vi "02 HEWH 24 Hour Test SM1.vi"(0 "Equipment":T5={"MW100"="MW100", "AG34970"="A-34972A", "WT210"="A-34972A"}, 2 "Semiphore":T6, 11 "Error In":errorcluster) -> (15 "Error Out":errorcluster)   [LabVIEW 2014]
uses:
  Type Definitions/ChannelSettings.ctl
  <vilib>/Utility/file.llb/Write To Spreadsheet File (string).vi
  Type Definitions/PowerElements.ctl
  Type Definitions/TestedFlowratesScenarios.ctl
  Type Definitions/Intellfaucet Mode.ctl
  Type Definitions/ValveBankPositions.ctl
  Type Definitions/HEWH Error Enumeration.ctl
  Support VIs/Global HEWH.vi
  <vilib>/Analysis/NI_AALBase.lvlib
  <vilib>/Analysis/baseanly.llb/Mean (DBL).vi
  Utility/Labview GEA2 Toolkit v2.1/library/GEA2_Toolkit.lvlib
  Type Definitions/EquipReferences.ctl
  Type Definitions/HEWH Tank Indicator.ctl
  <vilib>/Platform/fileVersionInfo.llb/FileVersionInformation.ctl
  Utility/GEA2 Commands/HEWH/Type Definitions/HEWH_Mode.ctl
  Utility/GEA2 Commands/HEWH/Type Definitions/WaterHeater GEA2 Data.ctl
  Utility/LabVIEW GEA2 Toolkit v2.0/type defs/Button Status.ctl
  Utility/GEA2 Commands/HEWH/Type Definitions/Status Query.ctl
  Utility/GEA2 Commands/HEWH/Type Definitions/Service Error Codes.ctl
panel:
  out "DrawCount 2":i32
  out "Dispense Schedule 2":dbl[](array[numeric])=[10.72, 10.72, 10.72, 10.72, 10.72, 10.72] format="%.2f"
  out "Loop":dbl
  out "deleted portion":dbl[](array[numeric])
  in  "Tab Control 3":enum32{"Page 1", "Page 2"}(tab)
  out "Water Heater GEA2 Data":T1 {"CRC" format="%x"; "Length" format="%x"; "Command" format="%x"; "Destination" format="%x"; "Source" format="%x"}
  in  "Tab Control":enum32{"Page 1", "Page 2"}(tab)
  in  "Time Reset":bool
  in  "Time Update":dbl format="%<%H:%M:%S>t"
  out "Tc Tree Check":dbl[](array[numeric]) format="%.4f"
  out "Serial Data In":string
  in  "IP Agilent":string="192.168.25.2"
  in  "IP MW100":string="192.168.25.4"
  out "Label Array":string[](array[string])
  out "Chanel List":string
  out "Computer Name":string
  in  "Stop Logging":bool
  in  "stop":bool
  out "StopSerial":bool
  out "FileVersionInfo Out":T7
  out "GEA2 Write Setpoints":errorcluster
  out "Calibration File Array":dbl[][](array[numeric])
  out "Flow Rate (GPM)":dbl
  out "Degrees F":dbl
  out "Voltage":dbl=240.0
  out "Number of Records":i32
  in  "Stop Test Seqence":bool
  out "Ver.":string
  out "Log Data":string[][](array[string])
  out "DrawCount":i32
  out "POWER":T8
  out "t*=0":dbl format="%<%H:%M:%S>t"
  out "Elapsed.Time (H:M:S)":dbl format="%<%H:%M:%S>t"
  out "STATUS":string
  in  "Help":bool
  out "Tank Display":T9 {"TC6" format="%.2g"; "TIN" format="%.2g"; "TOUT" format="%.2g"; "Mean" format="%.2f"; "Std Dev" format="%.2f"; "TC5" format="%.2g"; "TC4" format="%.2g"; "TC3" format="%.2g"; "TC2" format="%.2g"; "TC1" format="%.2g"}
  out "Current Draw Start Time":dbl format="%.2f"
  out "First Time":bool=TRUE
  out "Current State":string
  out "MW100":refnum<visa-resource-name>
  in  "Tab Control 2":enum32{"TEST STATUS", "DATA VIEW"}(tab)
  in  "Status Tabl":T10(tab)=enum."External Program Controls"
  in  "Read Config File":bool
  in  "RTDin to Downspout Offset":dbl
  in  "Power Off Time":dbl=82800.0 format="%<%H:%M>t"
  in  "End Log Duration":dbl=3600.0 format="%<%H:%M>t"
  in  "Config Filename":string="HEWH First Hour Rating.ini"
  in  "Num of PreDraws(0-3)":i32=1
  out "GEA2 HyperData":bool
  out "Data Array":string[][](array[string])
  in  "Expansion Tank?":bool
  out "Dispense Times":dbl[](array[numeric])=[0.0, 3600.0, 7200.0, 10800.0, 14400.0, 18000.0] format="%<%H:%M>t"
  out "Dispense Schedule":dbl[](array[numeric])=[10.72, 10.72, 10.72, 10.72, 10.72, 10.72] format="%.2f"
  out "Flow Rate Schedule":dbl[](array[numeric])=[3.0, 3.0, 3.0, 3.0, 3.0, 3.0] format="%.2f"
  out "Temperature Schedule":dbl[](array[numeric])=[58.0, 58.0, 58.0, 58.0, 58.0, 58.0] format="%.2f"
  in  "Cold Water Available?":bool=TRUE
  in  "T3":u32=500
  out "Local?":bool
  out "LAN IP Address":string="192.168.25.3"
  out "Init Complete":bool=TRUE
  in  "T1":u32=1000
  in  "T4":u32=30
  in  "T5":u32=50
  in  "Purge Guard Time(s)":dbl=360.0
  out "PowerON":bool=TRUE
  in  "Sample Per.(s)":dbl=5.0
  in  "Power Off Guard Time20s)":u32=20
  in  "Working File Directory":path=path "c:/work"
  in  "Save File Directory":path=path "c:/data"
  out "FileName":path
  out "Use Agilent?":bool
  out "GEA2 Set Mode":T11=enum."HighDemand"
  out "Set PointOut":u8=140
  in  "Calibration File":path=path "C:/work/CalibrationFile.csv"
  out "Calibration File?":bool
  in  "T2":u32=150
  out "Monitoring Temps Chart":T12(graph)
  out "Tcs 1-6":dbl[](array[numeric])
  in  "Purge Right Now":bool
  out "Downspount Flow":dbl(graph)
  out "Downspout Flow":dbl=3.8899999999999997
  out "Downspout Temp":dbl=76.8
  out "Temp Band(+/- F)":dbl=50.0
  out "Flow rate Adj":dbl=85.11482133995038
  out "Downspount Temp":dbl(graph)
  out "TempAdj":dbl
  out "Failed to Start Count":dbl
  in  "RTD Band":dbl=2.0
  in  "Skip Waiting for Cutout":bool
  in  "mean tank upper lim":dbl=140.0
  in  "meant tank lower lim":dbl=130.0
  out "Temp Range Err":bool=TRUE
  out "mean":dbl format="%0.2f"
  in  "Power Off Check Limit":dbl=20.0
  out "M*-1":dbl
  in  "Skip Waiting for Temp 3":bool
  out "Tcs 1-6, Ave. 3":dbl[](array[numeric])
  out "Temps Chart 2":T13(graph)
  in  "Temp Decline Hystersis":dbl=0.2
  out "T_Ave_Max":dbl
  out "T_Ave":dbl
  out "LastDraw":bool=TRUE
  out "T*Max":dbl
  out "Special Last Draw":bool
  out "Discard Last Draw":bool
  out "T*Ave":dbl
  out "T*min":dbl
  out "Volume(Gal.)":dbl
  in  "Flow Adj":dbl=3.0
  in  "Adj Time":dbl=3.0
  in  "K(0.1)":dbl=0.1
  out "TcDown":dbl
  out "Gal Target":dbl
  out "Drawing":bool=TRUE
  out "RTD Out":cluster{dbl, dbl}[](graph)
  out "Flowmeter":cluster{dbl, dbl}[](graph)
  in  "Skip Draw0":bool
  out "TcDown 0":dbl
  out "FlowMeter During Draw0":cluster{dbl, dbl}[](graph)
  out "RTD Out 0":cluster{dbl, dbl}[](graph)
  out "WattHours":dbl
  out "Total Gallons Drawn":dbl
  out "Error History":string[](array[string])
  out "Com History":string[](array[string])
  out "Test Data":dbl[][](array[numeric])
  out "Executaion Sequence":string[](array[string])
  out "Error Datalogging":errorcluster={"status"=TRUE, "code"=-1073807346, "source"="VISA Read in Gather Test Data.vi"}
  out "Gallons Chart":dbl(graph)
  out "Temps":T12(graph) caption="Waveform Chart"
  out "Watt Chart":T14(graph)
  # "24-HOUR RATING TEST"
  # "For Testing Purposes"
  # "Input HEWH Dispense Schedule. Standard Dispense time is 0-5 hours, 10.72 gallons/dispense @ 3 GPM and 58 Deg F."
  # "Wait for Cutout..."
  # "Input relays don't detect that UE or LE are on, and Power reading <\nCompressor LL (0.35 kW currently)"
  # "WAIT FOR TOP HEATER AND COMP OFF."
  # "T*max is max ave temp"
  # "Record output water temp after 15 secs, and at 5 sec intervals thereafter\nMonitor inlet water temp, must be 58 +/- 2 F\nTerminate draw when output temp = T*max -25F, record T*min"
  # "Terminate draw.  Record Tmin*, Tmax*, Tave* and M*"
  # "(For Last Draw, If after 30 sec, T< last tmin, stop and discard measurements, else continue)"
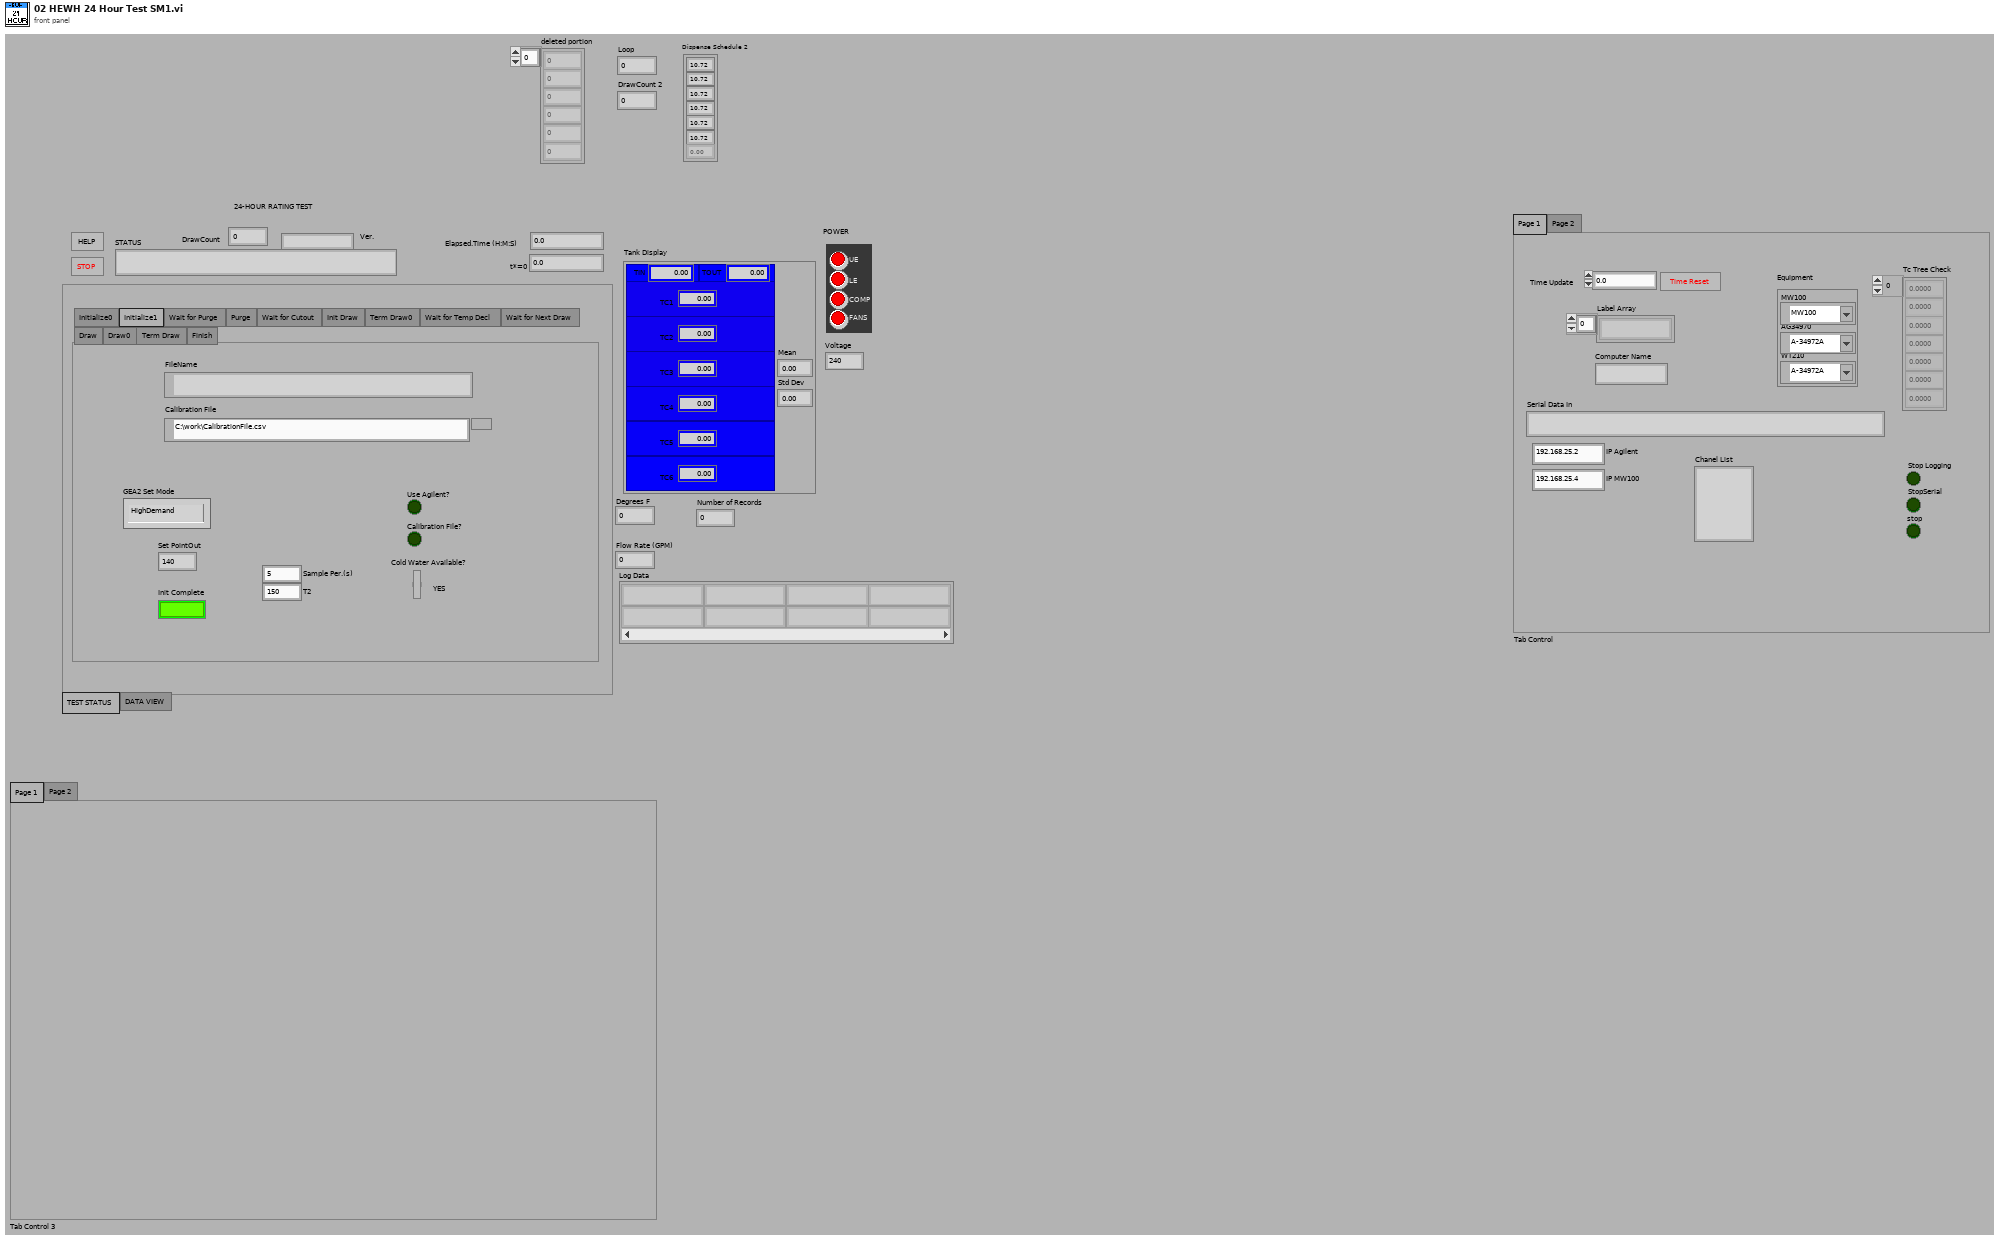
[diagram p1: front panel]
types:
  T1 = typedef "WaterHeater GEA2 Data.ctl" = cluster{"UE - state (1/0 on off)":u8, "LE - state (1/0 on off)":u8, "Comp - state (1/0 on off)":u8, "Fan  - state (1/0 on off)":u8, "Setpoint Deg F":i32, "T2(TankSensor)":dbl, "T3A(EvapIn)":dbl, "T3B(EvapOut)":dbl, "T4(CompressorDischarge)":dbl, "T5(Ambient)":dbl, "Current":dbl, "Voltage (Volts)":u16, "EEV Position (0-480)":u16, "Flow Events (Bit Encoded)":u16, "Heating Control Mode":u16, "Reason for last heating cycle termination":u16, "Reason Data word 1":string, "Reason Data word 2":string, "Reason Data word 3":string, "Reason Data word 4":string, "SW Debug Data":string, "Source":u8, "Destination":u8, "Command":u8, "Length":u8, "CRC":u16, "GEA2 Label Array":string[], " Critical Major SW Version (0-99)":u16, " Critical Minor SW Version (0-99)":u16, "Non Critical Major SW Version (0-99)":u16, "Non Critical Minor SW Version (0-99)":u16, "Software String":string, "GEA2 Data":string[], "Unit System Mode":string, "RQST_CURRENT_PID_SH_TARGET":u16, "RQST_DATA_FROM_DATA_FLASH":string, "RQST_DATA_FROM_Memory":string, "DSM Override Status":string, "IDLB_RESISTANCE":u32, "MODEL NUMBER":string, "MODEL_SELECT_AD_VALUE":u32, "RQST_OVERRIDE_STATUS":string, "PID_PARAMETERS":string[][], "READ_PERSONALITY":u8, "SERIAL_NUMBER":string, "SS_FAULT_COUNTS":string, "STD_ELEC_RANGE":string, "SUPPORTED_MODES":string[][], "T2 Resistance":u32, "T3B Resistance":u32, "T4 Resistance":u32, "T5 Resistance":u32, "Min Set Point (Deg F)":u32, "Max Set Point (Deg F)":u32, "Min Vacation Duration Days":u32, "Max Vacation Duration Days":u32, "Water Capacity (Gallons)":u32, "Button Status":T2, "Status Query":T3, "Service Error Codes":T4, "HEM_KWH_DATA":string[][], "OTHER_FAULT_COUNTS":string[][]}
  T2 = typedef "Button Status.ctl" = cluster{"Switch 1":bool, "Switch 2":bool, "Switch 3":bool, "Switch 4":bool, "Switch 5":bool, "Switch 6":bool, "Switch 7":bool, "Switch 8":bool, "Switch 9":bool, "Switch 10":bool, "Switch 11":bool, "Switch 12":bool, "Switch 13":bool, "Switch 14":bool, "Switch 15":bool, "Switch 16":bool}
  T3 = typedef "Status Query.ctl" = cluster{"Days Remaining (For Std Electric and Vacation)":u8, "Unit Status":string, "Current Tank Temp in Deg F":u8, "Current Setpoint in Deg F":u8, "Filter Status (% used)":u8, "Fallback Status (Fallback heating mode)":string, "Fallback Temp":u8, "\"Set Mode\" Selection":string}
  T4 = typedef "Service Error Codes.ctl" = cluster{"Reserved":bool, "Reserved 1":bool, "Reserved 2":bool, "Reserved 3":bool, "Reserved 4":bool, "Reserved 5":bool, "Reserved 6":bool, "Reserved 7":bool, "DataFlash Fail Status":bool, "Stuck Key Fail Status":bool, "Dry Tank Fail Status":bool, "Miswire Fail Status":bool, "Reserved 8":bool, "Reserved 9":bool, "Reserved 10":bool, "Reserved 11":bool, "UE Fail Status":bool, "LE Fail Status":bool, "Filter Fail Status":bool, "T3A Fail Status":bool, "T3B Fail Status":bool, "T4 Fail Status":bool, "T5 Fail Status":bool, "T2 Fail Status":bool, "SS Cond A Status":bool, "SS Cond B Status":bool, "SS Cond C Status":bool, "SS Cond D Status":bool, "SS Cond E Status":bool, "SS Cond F Status":bool, "SS Fan Status":bool, "CMP Fail Status":bool}
  T5 = typedef "EquipReferences.ctl" = cluster{"MW100":refnum<visa-resource-name>, "AG34970":refnum<visa-resource-name>, "WT210":refnum<visa-resource-name>}
  T6 = typedef "Semaphore RefNum" = refnum<k1>
  T7 = typedef "FileVersionInformation.ctl" = cluster{"FileVersion":string, "ProductName":string, "InternalName":string, "CompanyName":string, "LegalCopyright":string, "FileDescription":string}
  T8 = typedef "PowerElements.ctl" = cluster{"UE":bool, "LE":bool, "COMP":bool, "FANS":bool}
  T9 = typedef "HEWH Tank Indicator.ctl" = cluster{"TC1-D":bool, "TC2-D":bool, "TC3-D":bool, "TC4-D":bool, "TC5-D":bool, "RTD_IN":bool, "RTDOUT":bool, "TC1":dbl, "TC2":dbl, "TC3":dbl, "TC4":dbl, "TC5":dbl, "TIN":dbl, "TOUT":dbl, "Std Dev":dbl, "Mean":dbl, "TC6-D":bool, "TC6":dbl}
  T10 = enum32{"Initialize0", "External Program Controls", "External Program Controls 2", "Program Controls", "Feedback", "Init Draw", "Feedback 2", "Feedback 3", "Feedback 4", "Draw", "Draw0", "Feedback 5", "Feedback 6"}
  T11 = typedef "HEWH_Mode.ctl" = enum16{"Hybrid", "Std Electric", "eHeat", "HighDemand", "Vacation"}
  T12 = cluster{"Tc Tree[0]":dbl, "Tc Tree[1]":dbl, "Tc Tree[2]":dbl, "Tc Tree[3]":dbl, "Tc Tree[4]":dbl, "Tc Tree[5]":dbl}[]
  T13 = cluster{"[0]":dbl, "[1]":dbl, "[2]":dbl, "[3]":dbl, "[4]":dbl, "[5]":dbl, "[6]":dbl}[]
  T14 = cluster{"[0]":dbl, "[1]":dbl, "[2]":dbl, "[3]":dbl, "[4]":dbl, "[5]":dbl}[]
  T15 = typedef "Intellfaucet Mode.ctl" = enum16{"Adjust Temp", "Adjust Flow", "Start Flow", "Stop Flow"}
  T16 = typedef "ValveBankPositions.ctl" = enum16{"Heating", "Purge", "Resting", "Draw"}
  T17 = typedef "TestedFlowratesScenarios.ctl" = enum16{"DRK500,Station1", "DRK375,Lab", "SRK500,Station1,5GPM FR", "DRK375,STATION3,1/2\"HOSE", "DRK500,Station1,downspout", "DRK375,Station3,thruEcocute", "DRK375,Station3,purge", "Build2,2B,Purge", "Global, Purge", "Global, Tank", "DRK250"}
  T18 = typedef "HEWH Error Enumeration.ctl" = enum16{"No Error", "GEA2 Send ACK Mismatch", "GEA2 STX", "GEA2 ETX", "GEA2 CRC Mismatch", "GEA2 ReadACK", "RTD In Range Error", "Fail Mean Tank Temp", "No Flow Config Data Found", "Failed Flow During Purge", "Temp During Purge", "Confirm IF Stop Fail", "Init Draw: TC_1 Out of Range", "Flow = 0 During Draw after 20s"}
  T19 = enum16{"Computation Start", "Computation stop", "Reset Computation", "Clear Computation"}
  T20 = cluster{" Draw Test Condition":enum16{"DRK500,Station1", "DRK375,Lab", "SRK500,Station1,5GPM FR", "DRK500,Station1,downspout"}, "Serial Port Available?":bool, "Cold Water Available?":bool, "TempErLimit":dbl, "Temp Decline Hystersis":dbl, "Target IP Address":string}
  T21 = cluster{"Degree Setting":dbl, "Flow rate setting":dbl, "Tc1 LL":dbl, "Tc1 UL":dbl}
  T22 = cluster{"No Serial  Sample Period(s)":dbl, "T5":u32, "T4":u32, "T1":u32, "T2":u32, "T3":u32}
  T23 = typedef "Cluster Purge Settings.ctl" = cluster{"Temp SettleTimeLimit(S)":dbl, "Steady State Persist Time(mS)":u32, "Purge Min Time":i32, "Flow SettleTimeLimit(S)":dbl, "Flow Adjust Time (3s)":dbl, "Flow Band (+/-GPM)":dbl, "Proportional Control Adjust Rate":dbl}
  T24 = cluster{"PurgreTempLimit":dbl, "Purge Condition TC":enum16{"TC1", "TC2", "TC3", "TC4", "TC5", "TC6"}, "Purgre0TempLim":dbl, "Purge Guard Time(s)":dbl}
  T25 = typedef "GEA2_Toolkit.lvlib/Data In.ctl" = cluster{"Source":u8, "Destination":u8, "Command":u8, "Message":string}
  T26 = typedef "GEA2_Toolkit.lvlib/Data Out.ctl" = cluster{"Source":u8, "Destination":u8, "Command":u8, "Length":u8, "CRC":u16, "Message":string}
  T27 = typedef "Draw Pattern Setup.ctl" = cluster{"Dispense Times":dbl[], "Total Gallons Schedule":dbl[], "Flow Rate Schedule ":dbl[], "Incoming Water Temperature":dbl[], "PreDraw Pattern":dbl[][], "Repeat":bool, "24 Hour PreDraw":T28, "Draw Until?":bool[]}
  T28 = typedef "PreDraw.ctl" = enum16{"Zero Pre-Draws", "One Pre- Draws", "Two Pre-Draws", "Three Pre-Draws", ""}
  T29 = enum16{"Computation Start", "Computation stop", "Reset Computation", "Clear Computation"}[]
  T30 = cluster{"Tc Tree[0]":dbl, "Tc Tree[1]":dbl, "Tc Tree[2]":dbl, "Tc Tree[3]":dbl, "Tc Tree[4]":dbl, "Tc Tree[5]":dbl}
  T31 = cluster{"[0]":dbl, "[1]":dbl, "[2]":dbl, "[3]":dbl, "[4]":dbl, "[5]":dbl, "[6]":dbl}
  T32 = typedef "PowerData.ctl" = cluster{"Voltage (Volts)":dbl, "Current (Amps)":dbl, "Power (Watts)":dbl, "WattHours (Wh)":dbl, "TC Tree (AVG)":dbl, "Flow Rate (GPM)":dbl, "Gallons (Gal)":dbl, "RTD Out (Deg F)":dbl, "TC Down":dbl}
  T33 = typedef "ChannelSettings.ctl" = u32
  T34 = cluster{"[0]":dbl, "[1]":dbl, "[2]":dbl, "[3]":dbl, "[4]":dbl, "[5]":dbl}
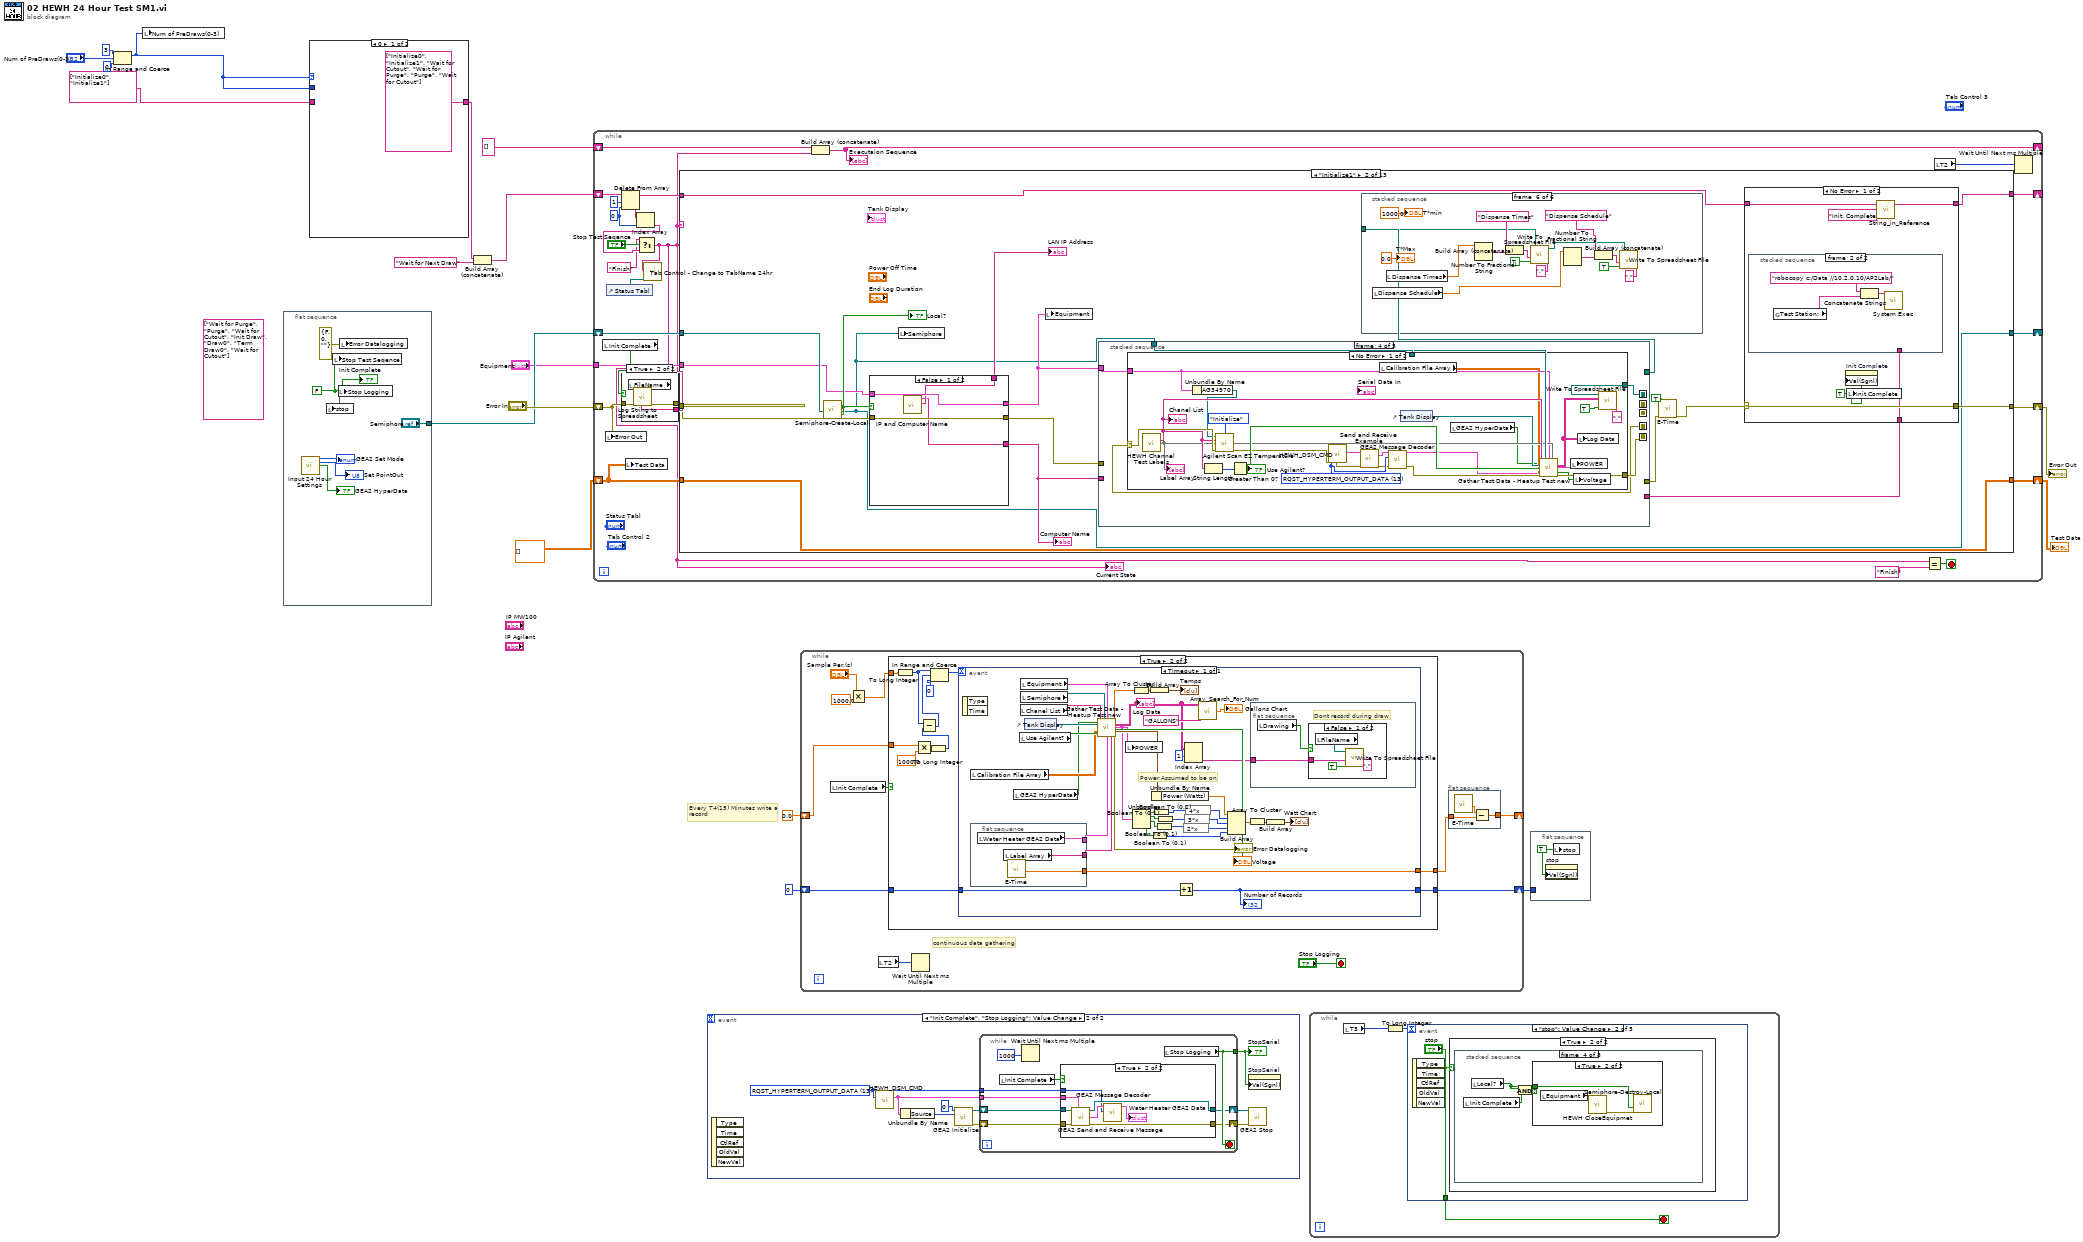
[diagram p0: block diagram]
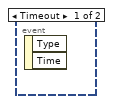
[diagram p2: hidden frame]
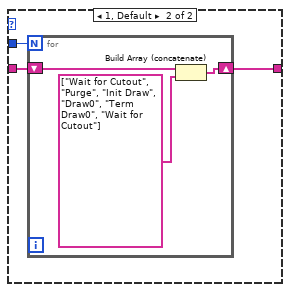
[diagram p4: hidden frame]
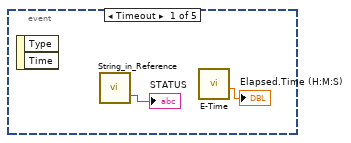
[diagram p5: hidden frame]
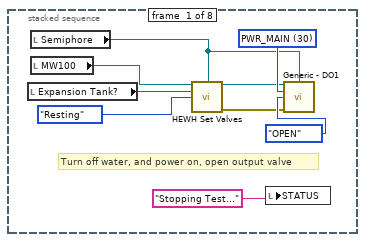
[diagram p7: hidden frame]
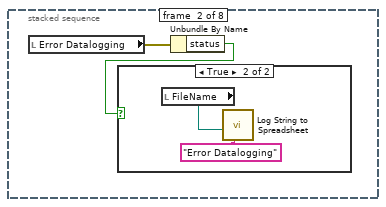
[diagram p8: hidden frame]
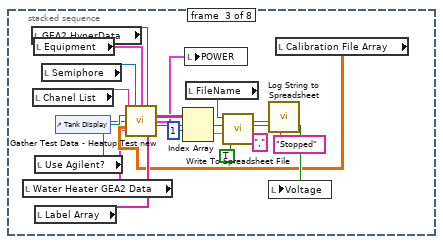
[diagram p10: hidden frame]
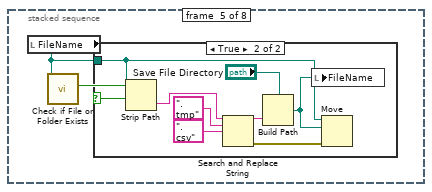
[diagram p12: hidden frame]
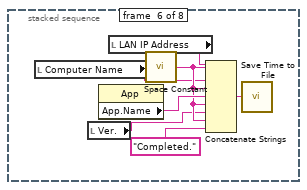
[diagram p14: hidden frame]
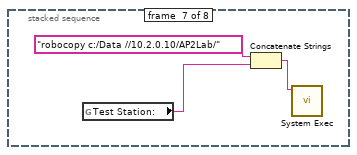
[diagram p15: hidden frame]
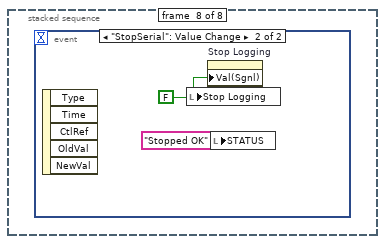
[diagram p16: hidden frame]
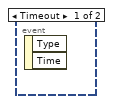
[diagram p17: hidden frame]
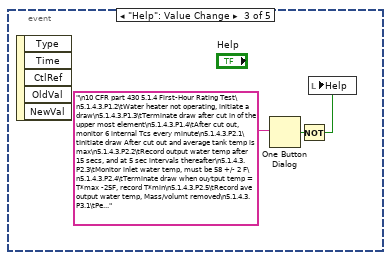
[diagram p18: hidden frame]
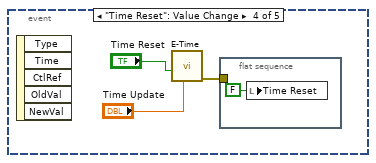
[diagram p19: hidden frame]
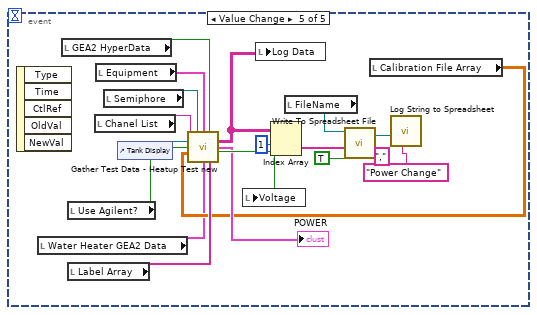
[diagram p20: hidden frame]
diagram:
  (unwired) string[] ["Wait for Purge", "Purge", "Wait for Cutout", "Init Draw", "Draw0", "Term Draw0", "Wait for Cutout"]
  # "Every T4(15) Minutes write a \nrecord"
  n1 = In Range and Coerce(upper limit=3, x="Num of PreDraws(0-3)", lower limit=0) -> (coerced(x)=w4:i32)  [unwired: 1 out]
  n2 = local write "Num of PreDraws(0-3)"(w4) -> ()
  n3 = flat-sequence {
    tunnel: ["Semiphore"] -> w16
    frame #0 {
      w23 = FALSE ("First Time 2")
      n4 = call "Input 24 Hour Settings.vi"() -> ("GEA2 Set Mode Out"=→"GEA2 Set Mode":T11, "Set PointOut"=→"Set PointOut":u8, "GEA2 HyperData Out"=→"GEA2 HyperData":bool)  [unwired: 12 in, 1 out]
      n5 = local write "stop"(w23) -> ()
      n6 = local write "Stop Test Seqence"(w23) -> ()
      n7 = local write "Stop Logging"(w23) -> ()
      n8 = local write "Error Datalogging"(errorcluster {"status"=FALSE, "code"=0, "source"=""} ("errordatalogging")) -> ()
      "Init Complete" <- w23
    }
  }
  n9 = case shown="0" w4 {
    tunnel: [string[] ["Initialize0", "Initialize1", "Wait for Cutout", "Wait for Purge", "Purge", "Wait for Cutout"] w28] -> w10
    tunnel: string[] ["Initialize0", "Initialize1"] -> [_ w27]
    tunnel: w4 -> [_ w26]
    frame 0 {
    }
    frame 1, Default {
      n10 = for {
        N: w26 -> [_]
        shift-right: [w29] -> w28
        shift-left: w27 -> [w31]
        n11 = Build Array (concatenate)(w31, string[] ["Wait for Cutout", "Purge", "Init Draw", "Draw0", "Term Draw0", "Wait for Cutout"]) -> (w29:string[])
      }
    }
  }
  n12 = Build Array (concatenate)(w10, "Wait for Next Draw") -> (w5:string[])
  n13 = while {
    shift-right: [w53] -> _
    shift-left: w5 -> [w56]
    shift-right: [w51] -> w17
    shift-left: "Error In" -> [w39]
    tunnel: "Equipment" -> [w47]
    shift-right: [w46] -> w14
    shift-left: dbl[][] [] -> [w45]
    shift-right: [w44] -> _
    shift-left: w16 -> [w48]
    shift-right: [w40] -> _
    shift-left: string[] [] -> [w41]
    stop <- w50 stop-if-true
    w43 = 0 ("index")
    n14 = local read "Init Complete"() -> (w37:bool)
    n15 = local write "Error Out"(w39) -> ()
    n16 = control-ref of="Status Tabl"() -> (w36:refnum<vi>)
    n17 = Delete From Array(array=w56, length=1, index=w43) -> (deleted portion=w54:string[], array with subset deleted=w52:string[])
    n18 = local write "Test Data"(w45) -> ()
    n19 = Index Array(array=w54, index=w43) -> (element=w34:string)
    n20 = Select(t="Finish" ("y"), s="Stop Test Seqence", f=w34) -> (s? t:f=w33:string)
    "Current State" <- w33
    n21 = case shown="True" w37 {
      tunnel: w39 -> [w57 w60]
      tunnel: [w57 w59] -> w38
      tunnel: w33 -> [_ w58]
      frame False {
      }
      frame True {
        n22 = local read "FileName"() -> (w61:path)
        n23 = call "Log String to Spreadsheet.vi"("String"=w58, "error in (no error)"=w60, "FileName"=w61) -> ("error out"=w59:errorcluster)  [unwired: 8 in]
      }
    }
    n24 = call "Tab Control - Change to TabName 24hr.vi"("Label.Text"=w33, "Status Tabl 3"=w36) -> ()  [unwired: 9 in]
    n25 = case shown="\"Initialize1\"" w33 {
      selector: w33 -> [_ _ _ _ _ _ _ _ _ _ _ _ w1179]
      tunnel: [w70 w113 w297 w375 w432 w553 w625 w691 w705 w886 w1028 w1145 w1194] -> w53
      tunnel: w52 -> [w70 w114 w298 w373 w430 w551 w626 w692 _ w887 w1028 w1146 w1193]
      tunnel: [w65 w111 w296 w374 w431 w552 w624 w690 w707 w884 w1029 w1144 w1180] -> w51
      tunnel: w38 -> [_ w112 w293 w366 w424 w536 w602 w688 w703 w888 w1026 w1117 w1181]
      tunnel: w48 -> [w71 w110 w300 w355 w428 w544 w607 w679 w704 w895 w1030 w1121 w1178]
      tunnel: w47 -> [_ w109 w299 w376 _ w543 _ _ _ w890 w1024 _ w1192]
      tunnel: [w72 w108 w301 w372 w429 w550 w627 w689 w706 w892 w1027 w1143 w1191] -> w46
      tunnel: w45 -> [w72 w108 w301 w372 w429 w550 w627 w689 w706 w892 w1027 w1142 w1191]
      tunnel: [w71 w101 w300 w355 w428 w544 w607 w679 w704 w891 w1025 w1121 w1178] -> w44
      frame "Initialize0" {
        w69 = FALSE ("Tool Bar:Show Abort Button")
        n26 = property class="VI"("TB.ShowAbortBut"=w69) -> ()  [unwired: 2 in, 2 out]
        n27 = property class="VI"("TB.ShowFreeRunBut"=w69) -> ()  [unwired: 2 in, 2 out]
        n28 = Current VI's Path() -> (path=w79:path)
        n29 = call "This VIs Path.vi"("path"=w79) -> ("current path"=w74:path, "File Version Info"=→"Ver.":string, "FileVersionInfo Out"=→"FileVersionInfo Out":T7, "error out"=w78:errorcluster)  [unwired: 10 in, 1 out]
        n30 = Build Path(base path=w74, name or relative path="Config Filename") -> (appended path=w77:path)
        n31 = case shown="False" "Read Config File" {
          tunnel: w77 -> [_ w88]
          tunnel: w78 -> [w80 w84]
          tunnel: [w80 w83] -> w66
          frame False {
          }
          frame True {
            n32 = call "Config File 24 Hour Test.vi"("Config File Path"=w88, "Error In"=w84) -> ("Test Condition Settings Cluster"=w87:T20, "DOE Test Spec Settings Cluster"=w86:T21, "Timing Cluster"=w85:T22, "Purge Settings Cluster"=w81:T23, "Purge Condition Settings Cluster"=w82:T24, "Error Out"=w83:errorcluster)  [unwired: 8 in]
            n33 = stacked-sequence {
              tunnel: w87 -> [w89 _ _ _ _ _]
              tunnel: w86 -> [_ w91 _ _ _ _]
              tunnel: w85 -> [_ _ w92 _ _ _]
              tunnel: [_ w90 _ _ _ _] -> _
              tunnel: w83 -> [_ _ _ _ _ w95]
              tunnel: w82 -> [_ _ _ _ w94 _]
              tunnel: w81 -> [_ _ _ w93 _ _]
              frame #0 {
                n34 = Unbundle(w89) -> ()  [unwired: 6 out]
              }
              frame #1 {
                n35 = Unbundle(w91) -> ("Flow rate setting"=w90:dbl)  [unwired: 3 out]
              }
              frame #2 {
                n36 = Unbundle(w92) -> ()  [unwired: 6 out]
              }
              frame #3 {
                n37 = Unbundle By Name(w93) -> ()  [unwired: 2 out]
              }
              frame #4 {
                n38 = Unbundle(w94) -> ()  [unwired: 4 out]
              }
              frame #5 {
                n39 = case shown="Error" w95 {
                  frame No Error {
                  }
                  frame Error {
                    n40 = call <vilib>:"Simple Error Handler.vi"("error in (no error)"=errorcluster {"status"=TRUE, "code"=-7600, "source"="Config File Error"}) -> ()  [unwired: 4 in, 5 out]
                    n41 = Stop(stop? (T)=TRUE) -> ()
                  }
                }
              }
            }
          }
        }
        n42 = call "String_in_Reference.vi"("String"="Initializing") -> ()  [unwired: 18 in, 1 out]
        n43 = call "Calibration File Check.vi"("error in (no error)"=w66, "Calibration Path"="Calibration File") -> ("error out"=w65:errorcluster, "Calibration File Array"=→"Calibration File Array":dbl[][], "Complete File?"=→"Calibration File?":bool)  [unwired: 6 in, 1 out]
      }
      frame "Initialize1" {
        n44 = call "Semiphore-Create-Local.vi"("Semiphore"=w110, "error in (no error)"=w112) -> ("semaphore"=w101:T6, "Local?"=w115:bool, "error out"=w116:errorcluster)  [unwired: 15 in]
        "Local?" <- w115
        n45 = case shown="False" w115 {
          tunnel: w116 -> [w280 w282]
          tunnel: [w279 w286] -> w104
          tunnel: [w280 w287] -> w103
          tunnel: w109 -> [w279 w281]
          tunnel: [w278 w284] -> w107
          tunnel: [w277 w283] -> w102
          frame False {
            n46 = call "IP and Computer Name.vi"() -> ("IP Address"=w278:string, "Computer Name"=w277:string)  [unwired: 10 in]
          }
          frame True {
            n47 = call "String_in_Reference.vi"("String"="INIT EQUIP") -> ()  [unwired: 18 in, 1 out]
            n48 = call "HEWH InitializeEquipmet.vi"("Error In"=w282, "Equipment"=w281) -> ("Error Out"=w287:errorcluster, 1:w283, 2:w284, "Equipment Out"=w286:T5)  [unwired: 6 in]
          }
        }
        "LAN IP Address" <- w107
        "Computer Name" <- w102
        n49 = local write "Semiphore"(w101) -> ()
        n50 = local write "Equipment"(w104) -> ()
        n51 = stacked-sequence {
          seq-local: [_ _ w174 _ _] -> [_ _ _ w186 _]
          seq-local: [_ w135 _ _ _] -> [_ _ w178 _ _]
          seq-local: [_ _ _ w188 _] -> [_ _ _ _ w220]
          seq-local: [_ w134 _ _ _] -> [_ _ _ w187 _]
          seq-local: [w119 _ _ _ _] -> [_ w139 _ _ _]
          tunnel: [_ _ _ _ w217] -> w99
          tunnel: w102 -> [_ w142 _ _ _]
          tunnel: w103 -> [w118 _ _ _ _]
          tunnel: w104 -> [_ _ w185 w190 w219]
          tunnel: w101 -> [_ _ w173 w189 _]
          tunnel: [_ w134 _ _ _] -> w100
          tunnel: [_ w146 _ _ _] -> w98
          frame #0 {
            # "Read globals.  Used in file init routine."
            n52 = local read "GEA2 HyperData"() -> (w117:bool)
            n53 = case shown="True" w117 {
              tunnel: [w120 w124] -> w119
              tunnel: w118 -> [w120 w126]
              frame False {
              }
              frame True {
                w122 = u8 15 items=["RQST_SOFTWARE_VERSION", "RQST_T2_RESISTANCE", "RQST_T3A_RESISTANCE", "RQST_T3B_RESISTANCE", "RQST_T4_RESISTANCE", "RQST_T5_RESISTANCE", "RQST_IDLB_RESISTANCE", "RQST_MODE_SELECT_RESISTANCE", "RQST_DATA_FROM_MEMORY", "RQST_DATA_FROM_DATA_FLASH", "RQST_SS_FAULT_COUNTS", "RQST_OTHER_FAULT_COUNTS", "CMD_CLEAR_FAULT_COUNTS", "RQST_HYPERTERM_OUTPUT_DATA", "CMD_RESET_FILTER_TIMES", "CMD_WRITE_SETPOINTS", "CMD_TURN_ON_OFF_DLB", "CMD_ENTER_EXIT_FCT_MODE", "CMD_SET_LEDS", "CMD_SET_EEV_DRIVE_LINES", "REQ_READ_KEY_STATUS", "RQST_READ_PERSONALITY", "CMD_ENTER_FACT_MODE", "CMD_RESET", "CMD_RESTORE_EEPROM_DEFAULTS", "CMD_SET_MODEL_NUMBER", "CMD_SET_SERIAL_NUMBER", "RQST_MODEL_NUMBER", "RQST_SERIAL_NUMBER", "CMD_TOGGLE_SERVICE_MODE", "CMD_TOGGLE_UE_SERV", "CMD_TOGGLE_LE_SERV", "CMD_REFRESH_SERVICE_TIMEOUTS", "RQST_DSM_OVERRIDE_STATUS", "RQST_STATUS_QUERY", "RQST_HEM_KWH_DATA", "RQST_SERVICE_ERROR_CODES", "RQST_OVERRIDE_STATUS", "CMD_UPDATE_DSM_LEVEL", "CMD_OVERRIDE_STATUS_CHANGED", "CMD_CLEAR_OVERRIDE_STATUS", "CMD_CLEAR_ENERGY_USAGE_CTRS", "CMD_DSM_OVERRIDES", "CMD_UPDATE_MODE", "CMD_SET_PID_P_DENOMINATOR", "CMD_SET_PID_I_DENOM_UNDER_THR", "CMD_SET_PID_I_DENOM_OVER_THR", "CMD_SET_START_POS_UNDER_THR", "CMD_SET_START_POS_OVER_THR", "CMD_SET_EEV_STOP_POSITION", "CMD_SET_AMBIENT_THRESH_1", "CMD_SET_AMBIENT_THRESH_2", "CMD_SET_AMBIENT_THRESH_3", "CMD_SET_PID_LOW_SH_TARGET", "CMD_SET_PID_MID_SH_TARGET", "RQST_PID_PARAMETERS", "CMD_COMP_OFF", "CMD_TOGGLE_FAN", "CMD_RQST_LED_STATUS", "CMD_UE_2_SECONDS", "CMD_LE_2_SECONDS", "CMD_COMP_ON", "CMD_HP_RUN_6MIN", "RQST_TEMP_RANGE", "RQST_VACATION_RANGE", "RQST_STD_ELEC_RANGE", "RQST_WATER_CAPACITY", "CMD_CANCEL_EEV_POSITION", "CMD_EEV_POSITION", "CMD_SET_CURRENTS", "RQST_SUPPORTED_MODES"] ("Command")
                w128 = u8 43 items=["RQST_SOFTWARE_VERSION", "RQST_T2_RESISTANCE", "RQST_T3A_RESISTANCE", "RQST_T3B_RESISTANCE", "RQST_T4_RESISTANCE", "RQST_T5_RESISTANCE", "RQST_IDLB_RESISTANCE", "RQST_MODE_SELECT_RESISTANCE", "RQST_DATA_FROM_MEMORY", "RQST_DATA_FROM_DATA_FLASH", "RQST_SS_FAULT_COUNTS", "RQST_OTHER_FAULT_COUNTS", "CMD_CLEAR_FAULT_COUNTS", "RQST_HYPERTERM_OUTPUT_DATA", "CMD_RESET_FILTER_TIMES", "CMD_WRITE_SETPOINTS", "CMD_TURN_ON_OFF_DLB", "CMD_ENTER_EXIT_FCT_MODE", "CMD_SET_LEDS", "CMD_SET_EEV_DRIVE_LINES", "REQ_READ_KEY_STATUS", "RQST_READ_PERSONALITY", "CMD_ENTER_FACT_MODE", "CMD_RESET", "CMD_RESTORE_EEPROM_DEFAULTS", "CMD_SET_MODEL_NUMBER", "CMD_SET_SERIAL_NUMBER", "RQST_MODEL_NUMBER", "RQST_SERIAL_NUMBER", "CMD_TOGGLE_SERVICE_MODE", "CMD_TOGGLE_UE_SERV", "CMD_TOGGLE_LE_SERV", "CMD_REFRESH_SERVICE_TIMEOUTS", "RQST_DSM_OVERRIDE_STATUS", "RQST_STATUS_QUERY", "RQST_HEM_KWH_DATA", "RQST_SERVICE_ERROR_CODES", "RQST_OVERRIDE_STATUS", "CMD_UPDATE_DSM_LEVEL", "CMD_OVERRIDE_STATUS_CHANGED", "CMD_CLEAR_OVERRIDE_STATUS", "CMD_CLEAR_ENERGY_USAGE_CTRS", "CMD_DSM_OVERRIDES", "CMD_UPDATE_MODE", "CMD_SET_PID_P_DENOMINATOR", "CMD_SET_PID_I_DENOM_UNDER_THR", "CMD_SET_PID_I_DENOM_OVER_THR", "CMD_SET_START_POS_UNDER_THR", "CMD_SET_START_POS_OVER_THR", "CMD_SET_EEV_STOP_POSITION", "CMD_SET_AMBIENT_THRESH_1", "CMD_SET_AMBIENT_THRESH_2", "CMD_SET_AMBIENT_THRESH_3", "CMD_SET_PID_LOW_SH_TARGET", "CMD_SET_PID_MID_SH_TARGET", "RQST_PID_PARAMETERS", "CMD_COMP_OFF", "CMD_TOGGLE_FAN", "CMD_RQST_LED_STATUS", "CMD_UE_2_SECONDS", "CMD_LE_2_SECONDS", "CMD_COMP_ON", "CMD_HP_RUN_6MIN", "RQST_TEMP_RANGE", "RQST_VACATION_RANGE", "RQST_STD_ELEC_RANGE", "RQST_WATER_CAPACITY", "CMD_CANCEL_EEV_POSITION", "CMD_EEV_POSITION", "CMD_SET_CURRENTS", "RQST_SUPPORTED_MODES"] ("Command")
                n54 = local read "GEA2 Set Mode"() -> (w127:T11)
                n55 = local read "Set PointOut"() -> (w121:u8)
                n56 = call "HEWH_DSM_CMD.vi"("Mode"=w127, "GEA2 Commands and Requests"=w128) -> ("Input Data"=w129:T25)  [unwired: 7 in, 1 out]
                n57 = call "Send Example.vi"("Input Data"=w129, "Error In"=w126) -> ("Error Out"=w125:errorcluster)  [unwired: 13 in]
                n58 = call "HEWH_DSM_CMD.vi"("Temperature"=w121, "GEA2 Commands and Requests"=w122) -> ("Input Data"=w123:T25)  [unwired: 7 in, 1 out]
                n59 = call "Send Example.vi"("Input Data"=w123, "Error In"=w125) -> ("Error Out"=w124:errorcluster)  [unwired: 13 in]
              }
            }
            "GEA2 Write Setpoints" <- w119
          }
          frame #1 {
            # "File init uses globals."
            # "Initialize Data file ."
            n60 = local read "FileVersionInfo Out"() -> (w144:T7)
            n61 = local read "GEA2 Set Mode"() -> (w131:T11)
            n62 = local read "Set PointOut"() -> (w136:u8)
            n63 = Unbundle By Name(w144) -> ("FileVersion"=w143:string)  [unwired: 1 out]
            n64 = case shown="\"Hybrid\", Default" w131 {
              tunnel: ["SE" ("Mode:") "EH" ("Mode:") "HD" ("Mode:") "HY" ("Mode:")] -> w132
              frame "Std Electric" {
              }
              frame "eHeat" {
              }
              frame "HighDemand" {
              }
              frame "Hybrid", Default {
              }
            }
            n65 = call "HEWH Data File Info String.vi"("Set PointOut"=w136, "GEA2 Set Mode"=w131) -> ("Info string"=w137:string)  [unwired: 9 in]
            n66 = local read "GEA2 HyperData"() -> (w130:bool)
            n67 = call "Data_File_Init.vi"("Data File Directory"="Working File Directory", "Test_Name In:"="24DOE", "Version In:"=w143, "Computer Name In:"=w142, "error in (no error)"=w139, "File Extension:"="tmp", "Ambient Temp / RH:"=w137, "Mode:"=w132) -> ("FileName"=w134:path, "Data Array"=w145:string[][], "error out"=w138:errorcluster)  [unwired: 5 in]
            "FileName" <- w134
            "Data Array" <- w145
            n68 = case shown="True" w130 {
              tunnel: w138 -> [w149 _]
              tunnel: [w149 w156] -> w135
              tunnel: w134 -> [_ w155]
              frame False {
              }
              frame True {
                w150 = u8 0 items=["RQST_SOFTWARE_VERSION", "RQST_T2_RESISTANCE", "RQST_T3A_RESISTANCE", "RQST_T3B_RESISTANCE", "RQST_T4_RESISTANCE", "RQST_T5_RESISTANCE", "RQST_IDLB_RESISTANCE", "RQST_MODE_SELECT_RESISTANCE", "RQST_DATA_FROM_MEMORY", "RQST_DATA_FROM_DATA_FLASH", "RQST_SS_FAULT_COUNTS", "RQST_OTHER_FAULT_COUNTS", "CMD_CLEAR_FAULT_COUNTS", "RQST_HYPERTERM_OUTPUT_DATA", "CMD_RESET_FILTER_TIMES", "CMD_WRITE_SETPOINTS", "CMD_TURN_ON_OFF_DLB", "CMD_ENTER_EXIT_FCT_MODE", "CMD_SET_LEDS", "CMD_SET_EEV_DRIVE_LINES", "REQ_READ_KEY_STATUS", "RQST_READ_PERSONALITY", "CMD_ENTER_FACT_MODE", "CMD_RESET", "CMD_RESTORE_EEPROM_DEFAULTS", "CMD_SET_MODEL_NUMBER", "CMD_SET_SERIAL_NUMBER", "RQST_MODEL_NUMBER", "RQST_SERIAL_NUMBER", "CMD_TOGGLE_SERVICE_MODE", "CMD_TOGGLE_UE_SERV", "CMD_TOGGLE_LE_SERV", "CMD_REFRESH_SERVICE_TIMEOUTS", "RQST_DSM_OVERRIDE_STATUS", "RQST_STATUS_QUERY", "RQST_HEM_KWH_DATA", "RQST_SERVICE_ERROR_CODES", "RQST_OVERRIDE_STATUS", "CMD_UPDATE_DSM_LEVEL", "CMD_OVERRIDE_STATUS_CHANGED", "CMD_CLEAR_OVERRIDE_STATUS", "CMD_CLEAR_ENERGY_USAGE_CTRS", "CMD_DSM_OVERRIDES", "CMD_UPDATE_MODE", "CMD_SET_PID_P_DENOMINATOR", "CMD_SET_PID_I_DENOM_UNDER_THR", "CMD_SET_PID_I_DENOM_OVER_THR", "CMD_SET_START_POS_UNDER_THR", "CMD_SET_START_POS_OVER_THR", "CMD_SET_EEV_STOP_POSITION", "CMD_SET_AMBIENT_THRESH_1", "CMD_SET_AMBIENT_THRESH_2", "CMD_SET_AMBIENT_THRESH_3", "CMD_SET_PID_LOW_SH_TARGET", "CMD_SET_PID_MID_SH_TARGET", "RQST_PID_PARAMETERS", "CMD_COMP_OFF", "CMD_TOGGLE_FAN", "CMD_RQST_LED_STATUS", "CMD_UE_2_SECONDS", "CMD_LE_2_SECONDS", "CMD_COMP_ON", "CMD_HP_RUN_6MIN", "RQST_TEMP_RANGE", "RQST_VACATION_RANGE", "RQST_STD_ELEC_RANGE", "RQST_WATER_CAPACITY", "CMD_CANCEL_EEV_POSITION", "CMD_EEV_POSITION", "CMD_SET_CURRENTS", "RQST_SUPPORTED_MODES"] ("Command")
                n69 = call "HEWH_DSM_CMD.vi"("GEA2 Commands and Requests"=w150) -> ("Input Data"=w154:T25)  [unwired: 8 in, 1 out]
                n70 = call "Send and Receive Example.vi"("Input Data"=w154) -> ("Coverted Data Out"=w153:T26)  [unwired: 12 in, 2 out]
                n71 = call "GEA2 Message Decoder.vi"("GEA2 Commands and Requests"=w150, "Coverted Data Out"=w153) -> ("Water Heater GEA2 Data"=w152:T1)  [unwired: 9 in]
                n72 = Unbundle By Name(w152) -> ("Software String"=w151:string)
                n73 = call "Log String to Spreadsheet.vi"("String"=w151, "FileName"=w155) -> ("error out"=w156:errorcluster)  [unwired: 9 in]
              }
            }
            n74 = Array To Spreadsheet String(delimiter (Tab)=",", array=w145, 3:"%s" ("format string")) -> (spreadsheet string=w146:string)
          }
          frame #2 {
            # "Solenoid Out+com port turns the com port off that controls the \ngallon calc. Turns off Gal Calc, initially."
            # "Set Valves."
            n75 = call "Dispense Schedule.vi"() -> ("Draw Patten Setup"=→"Dispense Times":T27, 6:→"Dispense Schedule", 8:w161, 10:w165)  [unwired: 11 in, 1 out]
            "Temperature Schedule" <- w165
            "Flow Rate Schedule" <- w161
            n76 = local read "DrawCount"() -> (w166:i32)
            n77 = Unbundle(w185) -> ("MW100"=w162:refnum<visa-resource-name>)  [unwired: 2 out]
            "MW100" <- w162
            n78 = Index Array(array=w165, index=w166) -> (element=→"Degrees F")
            n79 = Index Array(array=w161, index=w166) -> (element=→"Flow Rate (GPM)")
            n80 = call "HEWH Set Valves.vi"("VISA session"=w162, 2:w173, "Pressurize Tank?"="Expansion Tank?", "Valve Bank Setting"=ValveBankPositions."Heating", "Error In"=w178) -> ("dup VISA session"=w183:refnum<visa-resource-name>, "Error Out"=w182:errorcluster)  [unwired: 9 in]
            n81 = local read "Flow Rate (GPM)"() -> (w168:dbl)
            n82 = call "HEWH Totalize Flow Control.vi"("VISA session"=w183, 2:w173, "Totalize Flow"=FALSE, "error in (no error)"=w182) -> ("dup VISA session"=w176:refnum<visa-resource-name>, "error out"=w179:errorcluster)  [unwired: 10 in]
            n83 = call "Intellifaucet_Driver.vi"("VISA session"=w176, "Mode"=Intellfaucet_Mode."Adjust Flow", 2:w173, "Percent Flow"=w168, "Error In"=w179) -> ("VISA session out"=w171:refnum<visa-resource-name>, "Error Out"=w177:errorcluster)  [unwired: 9 in]
            n84 = local read "Degrees F"() -> (w167:dbl)
            n85 = call "Intellifaucet_Driver.vi"("VISA session"=w171, "Mode"=Intellfaucet_Mode."Adjust Temp", 2:w173, "Temperature(F)"=w167, "Error In"=w177) -> ("Error Out"=w174:errorcluster)  [unwired: 9 in, 1 out]
          }
          frame #3 {
            n86 = case shown="No Error" w186 {
              selector: w186 -> [w215 w216]
              tunnel: w190 -> [w207 _]
              tunnel: w189 -> [w210 _]
              tunnel: [w205 w216] -> w188
              tunnel: w187 -> [w201 _]
              frame No Error {
                w197 = u8 13 items=["RQST_SOFTWARE_VERSION", "RQST_T2_RESISTANCE", "RQST_T3A_RESISTANCE", "RQST_T3B_RESISTANCE", "RQST_T4_RESISTANCE", "RQST_T5_RESISTANCE", "RQST_IDLB_RESISTANCE", "RQST_MODE_SELECT_RESISTANCE", "RQST_DATA_FROM_MEMORY", "RQST_DATA_FROM_DATA_FLASH", "RQST_SS_FAULT_COUNTS", "RQST_OTHER_FAULT_COUNTS", "CMD_CLEAR_FAULT_COUNTS", "RQST_HYPERTERM_OUTPUT_DATA", "CMD_RESET_FILTER_TIMES", "CMD_WRITE_SETPOINTS", "CMD_TURN_ON_OFF_DLB", "CMD_ENTER_EXIT_FCT_MODE", "CMD_SET_LEDS", "CMD_SET_EEV_DRIVE_LINES", "REQ_READ_KEY_STATUS", "RQST_READ_PERSONALITY", "CMD_ENTER_FACT_MODE", "CMD_RESET", "CMD_RESTORE_EEPROM_DEFAULTS", "CMD_SET_MODEL_NUMBER", "CMD_SET_SERIAL_NUMBER", "RQST_MODEL_NUMBER", "RQST_SERIAL_NUMBER", "CMD_TOGGLE_SERVICE_MODE", "CMD_TOGGLE_UE_SERV", "CMD_TOGGLE_LE_SERV", "CMD_REFRESH_SERVICE_TIMEOUTS", "RQST_DSM_OVERRIDE_STATUS", "RQST_STATUS_QUERY", "RQST_HEM_KWH_DATA", "RQST_SERVICE_ERROR_CODES", "RQST_OVERRIDE_STATUS", "CMD_UPDATE_DSM_LEVEL", "CMD_OVERRIDE_STATUS_CHANGED", "CMD_CLEAR_OVERRIDE_STATUS", "CMD_CLEAR_ENERGY_USAGE_CTRS", "CMD_DSM_OVERRIDES", "CMD_UPDATE_MODE", "CMD_SET_PID_P_DENOMINATOR", "CMD_SET_PID_I_DENOM_UNDER_THR", "CMD_SET_PID_I_DENOM_OVER_THR", "CMD_SET_START_POS_UNDER_THR", "CMD_SET_START_POS_OVER_THR", "CMD_SET_EEV_STOP_POSITION", "CMD_SET_AMBIENT_THRESH_1", "CMD_SET_AMBIENT_THRESH_2", "CMD_SET_AMBIENT_THRESH_3", "CMD_SET_PID_LOW_SH_TARGET", "CMD_SET_PID_MID_SH_TARGET", "RQST_PID_PARAMETERS", "CMD_COMP_OFF", "CMD_TOGGLE_FAN", "CMD_RQST_LED_STATUS", "CMD_UE_2_SECONDS", "CMD_LE_2_SECONDS", "CMD_COMP_ON", "CMD_HP_RUN_6MIN", "RQST_TEMP_RANGE", "RQST_VACATION_RANGE", "RQST_STD_ELEC_RANGE", "RQST_WATER_CAPACITY", "CMD_CANCEL_EEV_POSITION", "CMD_EEV_POSITION", "CMD_SET_CURRENTS", "RQST_SUPPORTED_MODES"] ("Command")
                n87 = call "HEWH Channel Test Labels.vi"() -> ("Channel List"=w211:string, 8:w209)  [unwired: 12 in, 2 out]
                "Chanel List" <- w211
                "Label Array" <- w209
                n88 = Unbundle By Name(w207) -> ("AG34970"=w206:refnum<visa-resource-name>)
                n89 = String Length(string=w211) -> (length=w213:i32)
                n90 = call "Agilent Scan EZ Temperature.vi"("VISA Resource Name"=w206, "Control"=enum16{"Initialize", "Read", "Experiment"}."Initialize", "Channel Input"=w211, "error in (no error)"=w215) -> ("error out"=w194:errorcluster)  [unwired: 8 in, 3 out]
                n91 = Greater Than 0?(x=w213) -> (x > 0?=w212:bool)
                "Use Agilent?" <- w212
                n92 = call "HEWH_DSM_CMD.vi"("GEA2 Commands and Requests"=w197) -> ("Input Data"=w195:T25)  [unwired: 8 in, 1 out]
                n93 = call "Send and Receive Example.vi"("Input Data"=w195, "Error In"=w194) -> ("Coverted Data Out"=w196:T26, "Error Out"=w193:errorcluster)  [unwired: 11 in, 1 out]
                n94 = local read "Calibration File Array"() -> (w198:dbl[][])
                n95 = call "GEA2 Message Decoder.vi"("GEA2 Commands and Requests"=w197, "Coverted Data Out"=w196) -> ("Water Heater GEA2 Data"=w192:T1)  [unwired: 9 in]
                n96 = control-ref of="Tank Display"() -> (w200:refnum<vi>)
                n97 = local read "GEA2 HyperData"() -> (w191:bool)
                n98 = call "Gather Test Data - Heatup Test new.vi"("Power Analyzer"=w211, "GEA2?"=w210, "Equipment"=w207, "WT210 Current"=w191, "Tank Display Ref"=w200, "MW100 TC Headers"=w212, 9:"Calibration Coefficients"=w198, "error in (no error)"=w193, 13:"Calibration Coefficients"=w192, 14:w209) -> ("Output Data"=w202:string[][], "POWER"=w208:T8, "Read Mass Flow Rate"=w199:bool, "error out"=w205:errorcluster)  [unwired: 2 out]
                n99 = local write "POWER"(w208) -> ()
                n100 = local write "Voltage"(w199) -> ()
                n101 = local write "Log Data"(w202) -> ()
                n102 = call-poly <vilib>:"Write To Spreadsheet File.vi"("delimiter (\\t)"="," ("delimiter (\\t)"), "append to file? (new file:F)"=TRUE, "2D data"=w202, "file path (dialog if empty)"=w201) -> ()  [unwired: 4 in, 1 out]
              }
              frame Error {
              }
            }
          }
          frame #4 {
            w221 = T29 [enum."Computation Start", enum."Reset Computation"] items=["Computation Start", "Computation stop", "Reset Computation", "Clear Computation"]
            # "Reset and restart computation of gallons."
            n103 = Unbundle By Name(w219) -> ("MW100"=w218:refnum<visa-resource-name>)
            n104 = for {
              tunnel: w221 -> [w223] mode=indexing
              shift-right: [w224] -> w217
              shift-left: w220 -> [w225]
              tunnel: w218 -> [w222]
              n105 = call "YKMW100 Computation Control.vi"("VISA session"=w222, "Mode"=w223, "error in (no error)"=w225) -> ("error out"=w224:errorcluster)  [unwired: 11 in, 1 out]
            }
          }
        }
        n106 = stacked-sequence {
          tunnel: w100 -> [_ _ _ _ _ w247]
          frame #0 {
            # "Clear Charts."
            n107 = property on="Temps Chart 2" class="WFChart (strict)"("History Data"=T13 []) -> ()  [unwired: 2 in, 2 out]
            n108 = property on="Watt Chart" class="WFChart (strict)"("History Data"=T14 []) -> ()  [unwired: 2 in, 2 out]
            n109 = property on="Monitoring Temps Chart" class="WFChart (strict)"("History Data"=T12 []) -> ()  [unwired: 2 in, 2 out]
            n110 = property on="Temps" class="WFChart (strict)"("History Data"=T12 []) -> ()  [unwired: 2 in, 2 out]
            n111 = property on="Gallons Chart" class="WFChart (strict)"("History Data"=dbl[] []) -> ()  [unwired: 2 in, 2 out]
            "DrawCount" <- 0
          }
          frame #1 {
            # "Flow Loop Time"
            # "30 Second Delay between Samples thru test"
            # "UI Refresh Rate"
            # "Loop Delays, prevent overwork Machine"
            # "Sample Period for Decision Data"
            "t*=0" <- 0.0 ("t*=0")
          }
          frame #2 {
            w233 = dbl[] [] ("History Data")
            n112 = local write "Failed to Start Count"(0.0 ("Failed to Start Count")) -> ()
            n113 = local write "Power Off Guard Time20s)"(u32 20 ("Power Off Guard Time")) -> ()
            n114 = property on="Downspount Temp" class="WFChart (strict)"("History Data"=w233) -> ()  [unwired: 2 in, 2 out]
            n115 = property on="Downspount Flow" class="WFChart (strict)"("History Data"=w233) -> ()  [unwired: 2 in, 2 out]
          }
          frame #3 {
            w237 = TRUE ("First Time")
            w236 = FALSE ("BottomHeater")
            n116 = local write "Temp Range Err"(w236) -> ()
            n117 = local write "Drawing"(w236) -> ()
            n118 = local write "Skip Waiting for Cutout"(w236) -> ()
            n119 = local write "Purge Right Now"(w236) -> ()
            n120 = local write "Time Reset"(w236) -> ()
            n121 = local write "Skip Draw0"(w236) -> ()
            n122 = local write "LastDraw"(w236) -> ()
            n123 = local write "Help"(w236) -> ()
            n124 = local write "POWER"(T8 {"UE"=FALSE, "LE"=FALSE, "COMP"=FALSE, "FANS"=FALSE} ("POWER 2")) -> ()
            "First Time" <- w237
            "Special Last Draw" <- w236
            "Discard Last Draw" <- w236
            "PowerON" <- w237
          }
          frame #4 {
            n125 = Select(t="RTD Band", s="Cold Water Available?", f=55.0) -> (s? t:f=→"Temp Band(+/- F)":dbl)
          }
          frame #5 {
            n126 = local read "Dispense Schedule"() -> (w244:dbl[])
            n127 = local read "Dispense Times"() -> (w243:dbl[])
            n128 = Number To Fractional String(number=w243) -> (F-format string=w253:string[])  [unwired: 3 in]
            n129 = Build Array (concatenate)("Dispense Times" ("string"), w253) -> (w255:string[])
            n130 = call-poly <vilib>:"Write To Spreadsheet File.vi"("delimiter (\\t)"="," ("delimiter (\\t)"), "append to file? (new file:F)"=TRUE, "1D data"=w255, "file path (dialog if empty)"=w247) -> ("new file path (Not A Path if cancelled)"=w246:path)  [unwired: 4 in]
            n131 = Number To Fractional String(number=w244) -> (F-format string=w252:string[])  [unwired: 3 in]
            n132 = Build Array (concatenate)("Dispense Schedule" ("string"), w252) -> (w251:string[])
            n133 = call-poly <vilib>:"Write To Spreadsheet File.vi"("delimiter (\\t)"="," ("delimiter (\\t)"), "append to file? (new file:F)"=TRUE, "1D data"=w251, "file path (dialog if empty)"=w246) -> ()  [unwired: 4 in, 1 out]
            "T*Max" <- 0.0 ("T*Max")
            "T*min" <- 1000.0 ("T*min")
          }
        }
        n134 = call "E-Time.vi"("error in (no error)"=w99, "Reset"=TRUE) -> ("error out"=w105:errorcluster)  [unwired: 7 in, 2 out]
        n135 = case shown="No Error" w105 {
          selector: w105 -> [w263 w276]
          tunnel: [w262 string[] ["Finish"] ("States")] -> w113
          tunnel: [w263 w276] -> w111
          tunnel: w114 -> [w262 _]
          tunnel: w98 -> [w260 _]
          frame No Error {
            w259 = TRUE ("Init Complete")
            n136 = stacked-sequence {
              tunnel: w260 -> [w264 _]
              frame #0 {
                w268 = ","
                n137 = property class="App"() -> ("App.Name"=w267:string)  [unwired: 2 in, 2 out]
                n138 = local read "Computer Name"() -> (w271:string)
                n139 = local read "Ver."() -> (w270:string)
                n140 = local read "LAN IP Address"() -> (w266:string)
                n141 = Concatenate Strings(w266, w268, w271, w268, w267, w268, w270, w268, "Started. " ("string"), w264) -> (w265:string)
                n142 = call "Save Time to File.vi"("String"=w265) -> ()  [unwired: 13 in, 2 out]
              }
              frame #1 {
                n143 = global read "Global HEWH.vi" "Test Station:"() -> (w273:string)
                n144 = Concatenate Strings("robocopy c:/Data //10.2.0.10/AP2Lab/" ("command line"), w273) -> (w274:string)
                n145 = call <vilib>:"System Exec.vi"("command line"=w274) -> ()  [unwired: 7 in, 4 out]
              }
            }
            n146 = property on="Init Complete" class="Bool (strict)"("Val(Sgnl)"=w259) -> ()  [unwired: 2 in, 2 out]
            n147 = local write "Init Complete"(w259) -> ()
            n148 = call "String_in_Reference.vi"("String"="Init. Complete") -> ()  [unwired: 18 in, 1 out]
          }
          frame Error {
          }
        }
      }
      frame "Wait for Purge" {
        # "Purge with control, or drawcount=0 or error,\nor stop, or \ndispense time - current draw time > purge guard time."
        n149 = local read "Dispense Times"() -> (w291:dbl[])
        n150 = local read "DrawCount"() -> (w292:i32)
        n151 = Index Array(array=w291, index=w292) -> (element=w289:dbl)
        n152 = local read "t*=0"() -> (w290:dbl)
        n153 = while {
          tunnel: w300 -> [w347]
          shift-right: [w338] -> w295
          shift-left: w293 -> [w337]
          tunnel: w299 -> [w340]
          tunnel: " Purge Condition. NextDispenseTime-Elaspse time < Purge Guard Time. t =   " ("string") -> [w319]
          tunnel: w290 -> [w314]
          tunnel: w289 -> [w313]
          tunnel: "Purge Guard Time(s)" -> [w312]
          i -> [w321]
          stop <- w323 stop-if-true
          n154 = local read "DrawCount"() -> (w333:i32)
          n155 = local read "GEA2 HyperData"() -> (w307:bool)
          n156 = call "E-Time.vi"("error in (no error)"=w337) -> ("error out"=w336:errorcluster, "Elapsed Time (sec)"=w329:dbl)  [unwired: 8 in, 1 out]
          n157 = local read "Water Heater GEA2 Data"() -> (w308:T1)
          n158 = local read "Use Agilent?"() -> (w310:bool)
          n159 = local read "Label Array"() -> (w311:string[])
          n160 = local read "Chanel List"() -> (w326:string)
          n161 = control-ref of="Tank Display"() -> (w339:refnum<vi>)
          n162 = local read "Calibration File Array"() -> (w309:dbl[][])
          n163 = Equal To 0?(x=w333) -> (x = 0?=w332:bool)
          n164 = Compound Arithmetic op=unknown(w313, w314, invert w312) -> (w318:dbl)
          n165 = call "Gather Test Data - Heatup Test new.vi"("Power Analyzer"=w326, "GEA2?"=w347, "Equipment"=w340, "WT210 Current"=w307, "Tank Display Ref"=w339, "MW100 TC Headers"=w310, 9:"Calibration Coefficients"=w309, "error in (no error)"=w336, 13:"Calibration Coefficients"=w308, 14:w311) -> ("Tc Tree"=w335:dbl[], "Output Data"=w327:string[][], "POWER"=w315:T8, "Read Mass Flow Rate"=w320:bool, "error out"=w338:errorcluster)  [unwired: 1 out]
          "Tcs 1-6" <- w335
          n166 = local write "Voltage"(w320) -> ()
          n167 = Subtract(x=w313, y=w312) -> (x-y=w330:dbl)
          n168 = Number To Decimal String(number=w318) -> (decimal integer string=w317:string)  [unwired: 1 in]
          n169 = local write "Log Data"(w327) -> ()
          n170 = local write "POWER"(w315) -> ()
          n171 = Array To Cluster(array=w335) -> (cluster=w345:T30)
          n172 = Subtract(x=w329, y=w314) -> (x-y=w328:dbl)
          n173 = Build Array(w345) -> (→"Monitoring Temps Chart":T12)
          n174 = Greater?(x=w328, y=w330) -> (0:w325:bool)
          n175 = Number To Decimal String(number=w321) -> (decimal integer string=w341:string)  [unwired: 1 in]
          n176 = Equal To 0?(x=w321) -> (x = 0?=w322:bool)
          n177 = Unbundle By Name(w338) -> ("status"=w346:bool)
          n178 = local read "Stop Test Seqence"() -> (w316:bool)
          n179 = Concatenate Strings(w319, w317, w341, " Readings" ("string")) -> (w342:string)
          n180 = call "String_in_Reference.vi"("String"=w342) -> ()  [unwired: 18 in, 1 out]
          n181 = local read "T1"() -> (w334:u32)
          n182 = Compound Arithmetic op=OR(w316, w346, w325, "Purge Right Now", w332) -> (w323:bool)
          n183 = Compound Arithmetic op=OR(w322, w323) -> (w324:bool)
          n184 = case shown="True" w324 {
            tunnel: w327 -> [_ w349]
            frame False {
            }
            frame True {
              n185 = Index Array(array=w349, index (row)=1) -> (element=w348:string[])  [unwired: 1 in]
              n186 = local read "FileName"() -> (w353:path)
              n187 = call-poly <vilib>:"Write To Spreadsheet File.vi"("delimiter (\\t)"="," ("delimiter (\\t)"), "append to file? (new file:F)"=TRUE, "1D data"=w348, "file path (dialog if empty)"=w353) -> ()  [unwired: 4 in, 1 out]
            }
          }
          n188 = Wait (ms)(milliseconds to wait=w334) -> ()  [unwired: 1 out]
        }
        n189 = case shown="No Error" w295 {
          selector: w295 -> [w303 w306]
          tunnel: [w304 string[] ["Finish"] ("States")] -> w297
          tunnel: w298 -> [w304 _]
          tunnel: [w303 w306] -> w296
          frame No Error {
            # "Press it each time."
            n190 = local write "Purge Right Now"(FALSE ("Skip Waiting for Temp")) -> ()
          }
          frame Error {
          }
        }
      }
      frame "Purge" {
        n191 = flat-sequence {
          tunnel: [w389] -> w369
          tunnel: [w388] -> w368
          tunnel: [w393] -> w367
          frame #0 {
            n192 = local read "DrawCount"() -> (w387:i32)
            n193 = local read "DrawCount"() -> (w385:i32)
            n194 = local read "Temperature Schedule"() -> (w390:dbl[])
            n195 = local read "Flow Rate Schedule"() -> (w391:dbl[])
            n196 = Not Equal To 0?(x=w387) -> (x != 0?=w386:bool)
            n197 = case shown="True" w386 {
              tunnel: w385 -> [w394 w396]
              tunnel: [w394 w395] -> w384
              frame False {
              }
              frame True {
                n198 = Decrement(x=w396) -> (x-1=w395:i32)
              }
            }
            n199 = Index Array(array=w391, index=w384) -> (element=w389:dbl)
            n200 = Index Array(array=w390, index=w384) -> (element=w388:dbl)
            n201 = local write "Degrees F"(w388) -> ()
            n202 = local write "Flow Rate (GPM)"(w389) -> ()
            n203 = local read "Temp Band(+/- F)"() -> (w393:dbl)
            n204 = call "String_in_Reference.vi"("String"="PurgeBegins" ("string")) -> ()  [unwired: 18 in, 1 out]
          }
        }
        n205 = flat-sequence {
          tunnel: [TestedFlowratesScenarios."Build2,2B,Purge" ("Test Condition")] -> w362
          frame #0 {
            n206 = call "String_in_Reference.vi"("String"="Purge Sequence Start") -> ()  [unwired: 18 in, 1 out]
          }
        }
        n207 = control-ref of="Downspount Temp"() -> (w364:refnum<vi>)
        n208 = control-ref of="Downspount Flow"() -> (w377:refnum<vi>)
        n209 = call "Purge Water Sequence SM.vi"("Degree Setting"=w368, "Equipment"=w376, "Semiphore"=w355, "Flow rate setting"=w369, "Temp Band(+/- F)"=w367, "Error In"=w366, "Flow Chart Ref"=w377, "Temp Chart Ref"=w364, "Test Condition"=w362) -> ("Failed to Start Count"=w359:dbl, "Downspout Flow"=→"Downspout Flow":dbl, "Downspout Temp"=→"Downspout Temp":dbl, "Flow rate setting out"=→"Flow rate Adj":dbl, "Temp Setting Out"=→"TempAdj":dbl, "Error Out"=w361:errorcluster)  [unwired: 1 in]
        "Failed to Start Count" <- w359
        n210 = Greater Than 0?(x=w359) -> (x > 0?=w360:bool)
        n211 = case shown="True" w360 {
          tunnel: w361 -> [w402 w408]
          tunnel: [w402 w407] -> w354
          tunnel: w359 -> [_ w403]
          frame False {
          }
          frame True {
            n212 = Number To Decimal String(number=w403) -> (decimal integer string=w405:string)  [unwired: 1 in]
            n213 = local read "FileName"() -> (w409:path)
            n214 = Concatenate Strings("Failed to Start Count" ("string"), w405) -> (w404:string)
            n215 = call "Log String to Spreadsheet.vi"("String"=w404, "error in (no error)"=w408, "FileName"=w409) -> ("error out"=w407:errorcluster)  [unwired: 8 in]
          }
        }
        n216 = flat-sequence {
          tunnel: [w379] -> w357
          tunnel: w354 -> [w378]
          frame #0 {
            w381 = "PurgeComplete" ("string")
            n217 = local read "FileName"() -> (w380:path)
            n218 = call "Log String to Spreadsheet.vi"("String"=w381, "error in (no error)"=w378, "FileName"=w380) -> ("error out"=w379:errorcluster)  [unwired: 8 in]
            n219 = call "String_in_Reference.vi"("String"=w381) -> ()  [unwired: 18 in, 1 out]
          }
        }
        n220 = Unbundle By Name(w357) -> ("source"=w358:string)
        n221 = case shown="\"True\", Default" w358 {
          selector: w358 -> [_ w399]
          tunnel: w357 -> [w397 w400]
          tunnel: [w397 w398] -> w356
          frame "" {
          }
          frame "True", Default {
            # "Purge not stable case may\njust posts this warning."
            n222 = local read "FileName"() -> (w401:path)
            n223 = call "Log String to Spreadsheet.vi"("String"=w399, "error in (no error)"=w400, "FileName"=w401) -> ("error out"=w398:errorcluster)  [unwired: 8 in]
          }
        }
        n224 = case shown="No Error" w356 {
          selector: w356 -> [w410 w413]
          tunnel: [w411 string[] ["Finish"] ("States")] -> w375
          tunnel: w373 -> [w411 _]
          tunnel: [w410 w413] -> w374
          frame No Error {
          }
          frame Error {
          }
        }
      }
      frame "Wait for Cutout" {
        # "At the end of the recovery period following\nthe first draw, record the maximum mean\ntank temperature observed after cut-out,\nT¯\nmax, 1, and the energy consumed by an electric\nresistance, gas or oil-fired water heater,\nQr. For heat pump water heaters, the total\nelectrical energy consumed during the first\nrecovery by the heat pump (including compressor,\nfan, controls, pump, etc.) and, if applicable,\nby the resistive element(s) shall be\nrecorded as Qr."
        n225 = local read "Chanel List"() -> (w425:string)
        n226 = while {
          tunnel: w428 -> [w461]
          shift-right: [w455] -> w418
          shift-left: w424 -> [w462]
          tunnel: w425 -> [w450]
          tunnel: [w440] -> w422
          tunnel: [w439] -> w415
          tunnel: [w438] -> w414
          i -> [w447]
          stop <- w446 continue-if-true
          # "Cutout for 2 samples in row"
          n227 = local read "Calibration File Array"() -> (w435:dbl[][])
          n228 = local read "Water Heater GEA2 Data"() -> (w434:T1)
          n229 = local read "GEA2 HyperData"() -> (w433:bool)
          n230 = local read "Use Agilent?"() -> (w437:bool)
          n231 = local read "Label Array"() -> (w436:string[])
          n232 = control-ref of="Tank Display"() -> (w452:refnum<vi>)
          n233 = local read "Equipment"() -> (w453:T5)
          n234 = call "Gather Test Data - Heatup Test new.vi"("Power Analyzer"=w450, "GEA2?"=w461, "Equipment"=w453, "WT210 Current"=w433, "Tank Display Ref"=w452, "MW100 TC Headers"=w437, 9:"Calibration Coefficients"=w435, "error in (no error)"=w462, 13:"Calibration Coefficients"=w434, 14:w436) -> ("Tc Tree"=w439:dbl[], "Output Data"=w451:string[][], "POWER"=w459:T8, "Read Mass Flow Rate"=w445:bool, "error out"=w455:errorcluster)  [unwired: 1 out]
          "Tc Tree Check" <- w439
          n235 = Unbundle(w459) -> ("UE"=w456:bool, "LE"=w457:bool, "COMP"=w458:bool)  [unwired: 1 out]
          n236 = Number To Decimal String(number=w447) -> (decimal integer string=w463:string)  [unwired: 1 in]
          n237 = local write "Log Data"(w451) -> ()
          n238 = Equal To 0?(x=w447) -> (x = 0?=w448:bool)
          n239 = Compound Arithmetic op=OR(w456, w457, w458) -> (w443:bool)
          n240 = local write "Voltage"(w445) -> ()
          n241 = local write "POWER"(w459) -> ()
          n242 = local read "Stop Test Seqence"() -> (w444:bool)
          n243 = while {
            tunnel: w443 -> [w469]
            shift-right: [w470] -> w442
            shift-left: _ -> [w468]
            stop <- TRUE stop-if-true
            n244 = case shown="False" w469 {
              tunnel: [w473 0.0] -> w470
              tunnel: w468 -> [w472 _]
              frame False {
                n245 = Increment(x=w472) -> (x+1=w473:dbl)
              }
              frame True {
              }
            }
          }
          n246 = Concatenate Strings("WAIT FOR CUTOUT.  " ("String"), w463, " checks." ("string")) -> (w465:string)
          n247 = Unbundle By Name(w455) -> ("status"=w467:bool)
          n248 = call "String_in_Reference.vi"("String"=w465) -> ()  [unwired: 18 in, 1 out]
          n249 = Less Or Equal?(x=w442, y="Power Off Check Limit") -> (x <= y?=w440:bool)
          n250 = local read "T1"() -> (w460:u32)
          n251 = call-poly <vilib>:"Mean.vi"("X"=w439) -> ("mean"=w438:dbl)  [unwired: 1 out]
          "mean" <- w438
          n252 = Wait (ms)(milliseconds to wait=w460) -> ()  [unwired: 1 out]
          n253 = Compound Arithmetic op=AND(invert w467, w440, invert "Skip Waiting for Cutout", invert w444) -> (w446:bool)
          n254 = Compound Arithmetic op=OR(w448, invert w446) -> (w449:bool)
          n255 = case shown="True" w449 {
            tunnel: w451 -> [_ w475]
            frame False {
            }
            frame True {
              n256 = Index Array(array=w475, index (row)=1) -> (element=w476:string[])  [unwired: 1 in]
              n257 = local read "FileName"() -> (w480:path)
              n258 = call-poly <vilib>:"Write To Spreadsheet File.vi"("delimiter (\\t)"="," ("delimiter (\\t)"), "append to file? (new file:F)"=TRUE, "1D data"=w476, "file path (dialog if empty)"=w480) -> ()  [unwired: 4 in, 1 out]
            }
          }
        }
        n259 = Unbundle By Name(w418) -> ("status"=w417:bool)
        n260 = Select(t="Error" ("String"), s=w417, f="Skip" ("String")) -> (s? t:f=w420:string)
        n261 = local read "FileName"() -> (w427:path)
        n262 = Select(t=w420, s=w422, f="Cutout" ("String")) -> (s? t:f=w423:string)
        n263 = call "Log String to Spreadsheet.vi"("String"=w423, "error in (no error)"=w418, "FileName"=w427) -> ("error out"=w426:errorcluster)  [unwired: 8 in]
        n264 = case shown="No Error" w426 {
          selector: w426 -> [w482 w532]
          tunnel: [w485 string[] ["Finish"] ("States")] -> w432
          tunnel: w430 -> [w484 _]
          tunnel: [w483 w532] -> w431
          tunnel: w415 -> [w493 _]
          tunnel: w414 -> [w481 _]
          frame No Error {
            # "Press Each Time"
            n265 = local read "DrawCount"() -> (w490:i32)
            n266 = Index Array(array=w484, index=0) -> (element=w492:string)
            n267 = Equal?(x=w490, y=0) -> (x = y?=w487:bool)
            n268 = Equal?(x=w492, y="Wait for Next Draw") -> (x = y?=w488:bool)
            n269 = And(x=w488, y=w487) -> (x .and. y?=w486:bool)
            n270 = case shown="True" w486 {
              tunnel: w493 -> [_ _]
              tunnel: [w497 w504] -> w485
              tunnel: w484 -> [w497 w503]
              tunnel: [w496 w500] -> w483
              tunnel: w482 -> [w496 w499]
              tunnel: w481 -> [_ w498]
              frame False {
              }
              frame True {
                n271 = local read "Temp Range Err"() -> (w501:bool)
                n272 = In Range and Coerce(upper limit="mean tank upper lim", x=w498, lower limit="meant tank lower lim") -> (In Range?=w505:bool)  [unwired: 1 out]
                n273 = case shown="True" w505 {
                  tunnel: [w512 w530] -> w504
                  tunnel: w503 -> [w513 w530]
                  tunnel: string[] ["Wait for Purge", "Purge", "Wait for Cutout", "Init Draw", "Term Draw0"] -> [w511 _]
                  tunnel: w501 -> [w510 _]
                  tunnel: [w509 w529] -> w500
                  tunnel: w499 -> [w508 w529]
                  frame False {
                    n274 = case shown="False" w510 {
                      tunnel: w513 -> [w521 _]
                      tunnel: [w520 string[] ["Finish"]] -> w512
                      tunnel: w511 -> [w519 _]
                      tunnel: [w516 w527] -> w509
                      tunnel: w508 -> [w517 w524]
                      frame False {
                        n275 = local read "FileName"() -> (w514:path)
                        n276 = Build Array (concatenate)(w519, w521) -> (w520:string[])
                        n277 = call "Log String to Spreadsheet.vi"("String"="Error: Mean Tank Temp", "error in (no error)"=w517, "FileName"=w514) -> ("error out"=w516:errorcluster)  [unwired: 8 in]
                        "Temp Range Err" <- TRUE ("Next Time Fail")
                      }
                      frame True {
                        n278 = local read "FileName"() -> (w522:path)
                        n279 = call "Log String to Spreadsheet.vi"("String"="Fail: Mean Tank Temp", "error in (no error)"=w524, "FileName"=w522) -> ("error out"=w523:errorcluster)  [unwired: 8 in]
                        n280 = call "Error Bool Enumerator.vi"("Error Enum"=HEWH_Error_Enumeration."Fail Mean Tank Temp", "Error In"=w523) -> ("Error Out"=w527:errorcluster)  [unwired: 7 in]
                      }
                    }
                  }
                  frame True {
                  }
                }
              }
            }
            n281 = local write "Skip Waiting for Cutout"(FALSE ("Skip Waiting for Cutout")) -> ()
          }
          frame Error {
          }
        }
      }
      frame "Wait for Temp Decl" {
        n282 = local read "FileName"() -> (w534:path)
        n283 = Number To Fractional String(number="Temp Decline Hystersis") -> (F-format string=w538:string)  [unwired: 3 in]
        n284 = Concatenate Strings("Record each new Tave maximum.  Wating for Ave temp to decl by   " ("string"), w538, "degrees F." ("string")) -> (w533:string)
        n285 = call "Log String to Spreadsheet.vi"("String"=w533, "error in (no error)"=w536, "FileName"=w534) -> ("error out"=w535:errorcluster)  [unwired: 8 in]
        n286 = while {
          tunnel: w544 -> [w589]
          shift-right: [w578] -> w542
          shift-left: w535 -> [w588]
          tunnel: w543 -> [w579]
          shift-right: [w571] -> w541
          shift-left: _ -> [w575]
          tunnel: "Temp Decline Hystersis" -> [w562]
          i -> [w564]
          stop <- w563 stop-if-true
          n287 = local read "Calibration File Array"() -> (w556:dbl[][])
          n288 = local read "Water Heater GEA2 Data"() -> (w555:T1)
          n289 = local read "Use Agilent?"() -> (w558:bool)
          n290 = local read "GEA2 HyperData"() -> (w554:bool)
          n291 = local read "Label Array"() -> (w557:string[])
          n292 = control-ref of="Tank Display"() -> (w574:refnum<vi>)
          n293 = local read "Chanel List"() -> (w577:string)
          n294 = call "Gather Test Data - Heatup Test new.vi"("Power Analyzer"=w577, "GEA2?"=w589, "Equipment"=w579, "WT210 Current"=w554, "Tank Display Ref"=w574, "MW100 TC Headers"=w558, 9:"Calibration Coefficients"=w556, "error in (no error)"=w588, 13:"Calibration Coefficients"=w555, 14:w557) -> ("Tc Tree"=w584:dbl[], "Output Data"=w568:string[][], "POWER"=w567:T8, "Read Mass Flow Rate"=w561:bool, "error out"=w578:errorcluster)  [unwired: 1 out]
          n295 = Number To Decimal String(number=w564) -> (decimal integer string=w581:string)  [unwired: 1 in]
          n296 = local write "Voltage"(w561) -> ()
          n297 = local write "POWER"(w567) -> ()
          n298 = call-poly <vilib>:"Mean.vi"("X"=w584) -> ("mean"=w572:dbl)  [unwired: 1 out]
          "T_Ave" <- w572
          n299 = local write "Log Data"(w568) -> ()
          n300 = Max & Min(x=w575, y=w572) -> (max(x,y)=w571:dbl)  [unwired: 1 out]
          "T_Ave_Max" <- w571
          n301 = Build Array (concatenate)(w584, w572) -> (w569:dbl[])
          "Tcs 1-6, Ave. 3" <- w569
          n302 = Subtract(x=w571, y=w572) -> (x-y=w576:dbl)
          n303 = Concatenate Strings("Wating for Ave temp to decl.  " ("string"), w581, " Readings." ("string")) -> (w582:string)
          n304 = Array To Cluster(array=w569) -> (cluster=w585:T31)
          n305 = call "String_in_Reference.vi"("String"=w582) -> ()  [unwired: 18 in, 1 out]
          n306 = Equal To 0?(x=w564) -> (x = 0?=w565:bool)
          n307 = Build Array(w585) -> (→"Temps Chart 2":T13)
          n308 = Greater Or Equal?(x=w576, y=w562) -> (x >= y?=w587:bool)
          n309 = local read "Stop Test Seqence"() -> (w560:bool)
          n310 = Unbundle By Name(w578) -> ("status"=w586:bool)
          n311 = local read "T1"() -> (w559:u32)
          n312 = Compound Arithmetic op=OR(w586, w587, "Skip Waiting for Temp 3", w560) -> (w563:bool)
          n313 = Compound Arithmetic op=OR(w565, w563) -> (w566:bool)
          n314 = case shown="True" w566 {
            tunnel: w568 -> [_ w590]
            frame False {
            }
            frame True {
              n315 = Index Array(array=w590, index (row)=1) -> (element=w591:string[])  [unwired: 1 in]
              n316 = local read "FileName"() -> (w595:path)
              n317 = call-poly <vilib>:"Write To Spreadsheet File.vi"("delimiter (\\t)"="," ("delimiter (\\t)"), "append to file? (new file:F)"=TRUE, "1D data"=w591, "file path (dialog if empty)"=w595) -> ()  [unwired: 4 in, 1 out]
            }
          }
          n318 = Wait (ms)(milliseconds to wait=w559) -> ()  [unwired: 1 out]
        }
        n319 = Number To Fractional String(number=w541) -> (F-format string=w545:string)  [unwired: 3 in]
        n320 = local read "FileName"() -> (w549:path)
        n321 = Concatenate Strings("Ave Temp Declined. Max Ave Tank Temp = " ("String"), w545) -> (w547:string)
        n322 = call "Log String to Spreadsheet.vi"("String"=w547, "error in (no error)"=w542, "FileName"=w549) -> ("error out"=w548:errorcluster)  [unwired: 8 in]
        n323 = case shown="No Error" w548 {
          selector: w548 -> [w596 w599]
          tunnel: [w597 string[] ["Finish"] ("States")] -> w553
          tunnel: w551 -> [w597 _]
          tunnel: [w596 w599] -> w552
          frame No Error {
          }
          frame Error {
          }
        }
      }
      frame "Init Draw" {
        # "Dont totalize flow on draw0"
        # "Valve must\nclose all the way\nbefore start works."
        n324 = flat-sequence {
          tunnel: [w629] -> w603
          tunnel: w602 -> [w629]
          frame #0 {
            n325 = local write "Drawing"(TRUE) -> ()
          }
        }
        n326 = local read "DrawCount"() -> (w611:i32)
        n327 = call "E-Time.vi"("error in (no error)"=w603) -> ("error out"=w617:errorcluster, "Elapsed Time (sec)"=w616:dbl)  [unwired: 8 in, 1 out]
        "Current Draw Start Time" <- w616
        n328 = local read "MW100"() -> (w601:refnum<visa-resource-name>)
        n329 = Equal?(x=1, y=w611) -> (x = y?=w619:bool)
        n330 = case shown="False" w619 {
          tunnel: w617 -> [w654 w664]
          tunnel: [w637 w662] -> w615
          tunnel: w616 -> [w655 _]
          tunnel: w601 -> [w653 _]
          tunnel: [w636 w663] -> w614
          frame True {
            n331 = local read "Water Heater GEA2 Data"() -> (w631:T1)
            n332 = local read "GEA2 HyperData"() -> (w630:bool)
            n333 = local write "t*=0"(w655) -> ()
            n334 = call "YKMW100 Computation Control.vi"("VISA session"=w653, "Mode"=T19."Reset Computation", "error in (no error)"=w654) -> ("error out"=w641:errorcluster)  [unwired: 11 in, 1 out]
            n335 = local read "Use Agilent?"() -> (w635:bool)
            n336 = local read "Label Array"() -> (w634:string[])
            n337 = local read "Chanel List"() -> (w650:string)
            n338 = local read "Equipment"() -> (w639:T5)
            n339 = local read "Semiphore"() -> (w649:T6)
            n340 = control-ref of="Tank Display"() -> (w651:refnum<vi>)
            n341 = local read "Calibration File Array"() -> (w632:dbl[][])
            n342 = call "Gather Test Data - Heatup Test new.vi"("Power Analyzer"=w650, "GEA2?"=w649, "Equipment"=w639, "WT210 Current"=w630, "Tank Display Ref"=w651, "MW100 TC Headers"=w635, 9:"Calibration Coefficients"=w632, "error in (no error)"=w641, 13:"Calibration Coefficients"=w631, 14:w634) -> ("Output Data"=w636:string[][], "POWER"=w633:T8, "Read Mass Flow Rate"=w640:bool, "error out"=w638:errorcluster)  [unwired: 2 out]
            n343 = Index Array(array=w636, index (row)=1) -> (element=w646:string[])  [unwired: 1 in]
            n344 = local read "FileName"() -> (w643:path)
            n345 = local write "POWER"(w633) -> ()
            n346 = local write "Voltage"(w640) -> ()
            n347 = call-poly <vilib>:"Write To Spreadsheet File.vi"("delimiter (\\t)"="," ("delimiter (\\t)"), "append to file? (new file:F)"=TRUE, "1D data"=w646, "file path (dialog if empty)"=w643) -> ("new file path (Not A Path if cancelled)"=w642:path)  [unwired: 4 in]
            n348 = call "Log String to Spreadsheet.vi"("String"="START (t*0)", "error in (no error)"=w638, "FileName"=w642) -> ("error out"=w637:errorcluster)  [unwired: 8 in]
          }
          frame False {
            n349 = local read "Water Heater GEA2 Data"() -> (w657:T1)
            n350 = local read "GEA2 HyperData"() -> (w656:bool)
            n351 = local read "Use Agilent?"() -> (w661:bool)
            n352 = local read "Chanel List"() -> (w673:string)
            n353 = local read "Label Array"() -> (w660:string[])
            n354 = local read "Equipment"() -> (w665:T5)
            n355 = local read "Semiphore"() -> (w672:T6)
            n356 = control-ref of="Tank Display"() -> (w674:refnum<vi>)
            n357 = local read "Calibration File Array"() -> (w658:dbl[][])
            n358 = call "Gather Test Data - Heatup Test new.vi"("Power Analyzer"=w673, "GEA2?"=w672, "Equipment"=w665, "WT210 Current"=w656, "Tank Display Ref"=w674, "MW100 TC Headers"=w661, 9:"Calibration Coefficients"=w658, "error in (no error)"=w664, 13:"Calibration Coefficients"=w657, 14:w660) -> ("Output Data"=w663:string[][], "POWER"=w659:T8, "Read Mass Flow Rate"=w666:bool, "error out"=w662:errorcluster)  [unwired: 2 out]
            n359 = local write "Voltage"(w666) -> ()
            n360 = local write "POWER"(w659) -> ()
            n361 = Index Array(array=w663, index (row)=1) -> (element=w669:string[])  [unwired: 1 in]
            n362 = local read "FileName"() -> (w667:path)
            n363 = call-poly <vilib>:"Write To Spreadsheet File.vi"("delimiter (\\t)"="," ("delimiter (\\t)"), "append to file? (new file:F)"=TRUE, "1D data"=w669, "file path (dialog if empty)"=w667) -> ()  [unwired: 4 in, 1 out]
          }
        }
        n364 = local write "Log Data"(w614) -> ()
        n365 = call "Array_Search_For_Num.vi"("N Rows of Data"=w614, "Title?"="GALLONS") -> ("number"=→"M*-1":dbl)  [unwired: 12 in, 1 out]
        n366 = Number To Fractional String(number=w611) -> (F-format string=w620:string)  [unwired: 3 in]
        n367 = local read "FileName"() -> (w623:path)
        n368 = Concatenate Strings("Drawcount = " ("string"), w620) -> (w622:string)
        n369 = call "Log String to Spreadsheet.vi"("String"=w622, "error in (no error)"=w615, "FileName"=w623) -> ("error out"=w600:errorcluster)  [unwired: 8 in]
        n370 = local read "Expansion Tank?"() -> (w606:bool)
        n371 = Not Equal To 0?(x=w611) -> (x != 0?=w610:bool)
        n372 = call "HEWH Set Valves.vi"("VISA session"=w601, 2:w607, "Pressurize Tank?"=w606, "Valve Bank Setting"=ValveBankPositions."Draw", "Error In"=w600) -> ("dup VISA session"=w609:refnum<visa-resource-name>, "Error Out"=w608:errorcluster)  [unwired: 9 in]
        n373 = call "HEWH Totalize Flow Control.vi"("VISA session"=w609, 2:w607, "Totalize Flow"=w610, "error in (no error)"=w608) -> ("error out"=w604:errorcluster)  [unwired: 10 in, 1 out]
        n374 = case shown="No Error" w604 {
          selector: w604 -> [w675 w678]
          tunnel: [w676 string[] ["Finish"] ("States")] -> w625
          tunnel: w626 -> [w676 _]
          tunnel: [w675 w678] -> w624
          frame No Error {
          }
          frame Error {
          }
        }
      }
      frame "Term Draw0" {
        # "The draw may be terminated anytime after\ncut-in occurs."
        n375 = flat-sequence {
          tunnel: w688 -> [w693]
          tunnel: [w693] -> w685
          frame #0 {
            (unwired) T12 [] ("History Data")
          }
        }
        n376 = local read "FileName"() -> (w687:path)
        n377 = call "Log String to Spreadsheet.vi"("String"="Term Draw 0", "error in (no error)"=w685, "FileName"=w687) -> ("error out"=w683:errorcluster)  [unwired: 8 in]
        n378 = local read "Expansion Tank?"() -> (w681:bool)
        n379 = local read "MW100"() -> (w680:refnum<visa-resource-name>)
        n380 = call "HEWH Set Valves.vi"("VISA session"=w680, 2:w679, "Pressurize Tank?"=w681, "Valve Bank Setting"=ValveBankPositions."Heating", "Error In"=w683) -> ("Error Out"=w682:errorcluster)  [unwired: 9 in, 1 out]
        n381 = case shown="No Error" w682 {
          selector: w682 -> [w694 w698]
          tunnel: [w695 string[] ["Finish"] ("States")] -> w691
          tunnel: w692 -> [w695 _]
          tunnel: [w694 w698] -> w690
          frame No Error {
          }
          frame Error {
            # "Press Each Time"
            n382 = local write "Skip Draw0"(FALSE ("Skip Draw0")) -> ()
          }
        }
      }
      frame "Wait for Next Draw" {
        # "When out of draws, waits for power off time, and turns off the power.  Then waits for finish time and finishes."
        # "Assumes Purging complete, and waiting on Time trigger."
        n383 = local read "Dispense Schedule"() -> (w702:dbl[])
        n384 = local read "DrawCount"() -> (w700:i32)
        n385 = Array Size(array=w702) -> (size(s)=w699:i32)
        n386 = Greater?(x=w699, y=w700) -> (0:w701:bool)
        n387 = case shown="True" w701 {
          tunnel: w704 -> [w714 _]
          tunnel: [w713 w848] -> w707
          tunnel: w703 -> [w710 w842]
          tunnel: [w715 w849] -> w705
          tunnel: w699 -> [_ w844]
          frame False {
            w708 = "Wait for Test Complete" ("String")
            n388 = local read "FileName"() -> (w711:path)
            n389 = local read "PowerON"() -> (w712:bool)
            n390 = call "Log String to Spreadsheet.vi"("String"=w708, "error in (no error)"=w710, "FileName"=w711) -> ("error out"=w709:errorcluster)  [unwired: 8 in]
            n391 = call "String_in_Reference.vi"("String"=w708) -> ()  [unwired: 18 in, 1 out]
            n392 = case shown="False" w712 {
              tunnel: [string[] ["Finish"] ("States") string[] ["Wait for Next Draw"] ("States")] -> w715
              tunnel: w709 -> [w747 w783]
              tunnel: w714 -> [w741 _]
              tunnel: [w724 w781] -> w713
              frame False {
                # "At 24 hours, record the\nmean tank temperature, T¯ 24, and the electric\nand/or fuel instrument readings."
                n393 = while {
                  tunnel: w747 -> [w757]
                  tunnel: [w756] -> w742
                  stop <- w750 stop-if-true
                  # "Wait for Finish Time."
                  n394 = local read "End Log Duration"() -> (w754:dbl)
                  n395 = local read "Power Off Time"() -> (w755:dbl)
                  n396 = local read "Stop Test Seqence"() -> (w749:bool)
                  n397 = local read "t*=0"() -> (w758:dbl)
                  n398 = call "E-Time.vi"("error in (no error)"=w757) -> ("error out"=w756:errorcluster, "Elapsed Time (sec)"=w760:dbl)  [unwired: 8 in, 1 out]
                  n399 = local read "T1"() -> (w752:u32)
                  n400 = Add(x=w754, y=w755) -> (x+y=w753:dbl)
                  n401 = Subtract(x=w760, y=w758) -> (x-y=w759:dbl)
                  n402 = Greater Or Equal?(x=w759, y=w753) -> (x >= y?=w751:bool)
                  n403 = Or(x=w751, y=w749) -> (x .or. y?=w750:bool)
                  n404 = Wait (ms)(milliseconds to wait=w752) -> ()  [unwired: 1 out]
                }
                n405 = local read "Water Heater GEA2 Data"() -> (w717:T1)
                n406 = local read "Calibration File Array"() -> (w718:dbl[][])
                n407 = local read "Use Agilent?"() -> (w720:bool)
                n408 = local read "Label Array"() -> (w719:string[])
                n409 = local read "Chanel List"() -> (w726:string)
                n410 = local read "Equipment"() -> (w744:T5)
                n411 = control-ref of="Tank Display"() -> (w743:refnum<vi>)
                n412 = local read "GEA2 HyperData"() -> (w716:bool)
                n413 = call "Gather Test Data - Heatup Test new.vi"("Power Analyzer"=w726, "GEA2?"=w741, "Equipment"=w744, "WT210 Current"=w716, "Tank Display Ref"=w743, "MW100 TC Headers"=w720, 9:"Calibration Coefficients"=w718, "error in (no error)"=w742, 13:"Calibration Coefficients"=w717, 14:w719) -> ("Tc Tree"=w739:dbl[], "Output Data"=w729:string[][], "POWER"=w727:T8, "PowerData"=w740:T32, "Read Mass Flow Rate"=w721:bool, "error out"=w731:errorcluster)
                n414 = Unbundle By Name(w740) -> ("WattHours (Wh)"=w733:dbl)
                n415 = local write "Voltage"(w721) -> ()
                n416 = call-poly <vilib>:"Mean.vi"("X"=w739) -> ("mean"=w738:dbl)  [unwired: 1 out]
                n417 = local write "POWER"(w727) -> ()
                n418 = Index Array(array=w729, index (row)=1) -> (element=w728:string[])  [unwired: 1 in]
                n419 = Number To Decimal String(number=w738) -> (decimal integer string=w737:string)  [unwired: 1 in]
                n420 = Number To Decimal String(number=w733) -> (decimal integer string=w732:string)  [unwired: 1 in]
                n421 = local read "FileName"() -> (w722:path)
                n422 = local write "Log Data"(w729) -> ()
                n423 = call-poly <vilib>:"Write To Spreadsheet File.vi"("delimiter (\\t)"="," ("delimiter (\\t)"), "append to file? (new file:F)"=TRUE, "1D data"=w728, "file path (dialog if empty)"=w722) -> ()  [unwired: 4 in, 1 out]
                n424 = Concatenate Strings("Measured at Tfinal: Tank Ave Temp = " ("String"), w737, ", Watts Hours = " ("String"), w732) -> (w735:string)
                n425 = call "Log String to Spreadsheet.vi"("String"=w735, "error in (no error)"=w731, "FileName"=w722) -> ("error out"=w725:errorcluster)  [unwired: 8 in]
                n426 = call "Log String to Spreadsheet.vi"("String"="Test Complete", "error in (no error)"=w725, "FileName"=w722) -> ("error out"=w724:errorcluster)  [unwired: 8 in]
              }
              frame True {
                w789 = T33 30 items=["4-20_OUT", "Pres_HI1", "Pres_HI2", "Pres_LOW", "Pres_PIN", "HEATER_TOP", "HEATER_BOT", "T_Shell", "FLOWMETER", "WATT_SENSE", "WH_TICK", "Tc_1", "Tc_2", "Tc_3", "Tc_4", "Tc_5", "Tc_6", "Tc_down", "T_Shell_2", "T_Shell_3", "T_Shell_4", "RTD_IN", "RTD_OUT", "RTD_AMB", "INTF_TEMPFLO", "INTF_READY", "INTF_START", "INTF_STOP", "DRM_LOW", "DRM_HIGH", "PWR_MAIN", "VLV_DUMP", "VLV_OUT", "VLV_IN", "WATT_HOURS", "FLOW(SAMPLE)", "GALLONS", "FLOW(GPM)"] ("Channel_Enum")
                # "Delay Long enough for last \nserial communication data acq to \ncomplete then Turn Off Power"
                n427 = local read "FileName"() -> (w793:path)
                n428 = call "Log String to Spreadsheet.vi"("String"="Wait for final Cutoff", "error in (no error)"=w783, "FileName"=w793) -> ("error out"=w794:errorcluster)  [unwired: 8 in]
                n429 = while {
                  tunnel: "Power Off Guard Time20s)" -> [w805]
                  shift-right: [w807] -> w782
                  shift-left: w794 -> [w812]
                  stop <- w800 stop-if-true
                  n430 = local read "Power Off Time"() -> (w806:dbl)
                  n431 = call "E-Time.vi"("error in (no error)"=w812) -> ("error out"=w807:errorcluster, "Elapsed Time (sec)"=w810:dbl)  [unwired: 8 in, 1 out]
                  n432 = local read "t*=0"() -> (w809:dbl)
                  n433 = call "String_in_Reference.vi"("String"="Wait for power off Time.") -> ()  [unwired: 18 in, 1 out]
                  n434 = local read "Stop Test Seqence"() -> (w802:bool)
                  n435 = local read "T1"() -> (w808:u32)
                  n436 = Subtract(x=w810, y=w809) -> (x-y=w811:dbl)
                  n437 = Subtract(x=w806, y=w805) -> (x-y=w804:dbl)
                  n438 = Wait (ms)(milliseconds to wait=w808) -> ()  [unwired: 1 out]
                  n439 = Greater?(x=w811, y=w804) -> (0:w801:bool)
                  n440 = Compound Arithmetic op=OR(w801, w802) -> (w800:bool)
                }
                n441 = local read "Chanel List"() -> (w775:string)
                n442 = local read "Semiphore"() -> (w792:T6)
                n443 = expression code="1000*x"("Power Off Guard Time20s)") -> (w769:u32)
                n444 = while {
                  tunnel: w792 -> [w831]
                  tunnel: w775 -> [w825]
                  tunnel: w782 -> [w829]
                  tunnel: [w828] -> w772
                  i -> [w821]
                  stop <- w820 continue-if-true
                  n445 = local read "Water Heater GEA2 Data"() -> (w814:T1)
                  n446 = local read "Calibration File Array"() -> (w815:dbl[][])
                  n447 = local read "GEA2 HyperData"() -> (w813:bool)
                  n448 = local read "Use Agilent?"() -> (w817:bool)
                  n449 = control-ref of="Tank Display"() -> (w824:refnum<vi>)
                  n450 = local read "Label Array"() -> (w816:string[])
                  n451 = local read "T1"() -> (w830:u32)
                  n452 = local read "Equipment"() -> (w832:T5)
                  n453 = call "Gather Test Data - Heatup Test new.vi"("Power Analyzer"=w825, "GEA2?"=w831, "Equipment"=w832, "WT210 Current"=w813, "Tank Display Ref"=w824, "MW100 TC Headers"=w817, 9:"Calibration Coefficients"=w815, "error in (no error)"=w829, 13:"Calibration Coefficients"=w814, 14:w816) -> ("Output Data"=w827:string[][], "POWER"=w826:T8, "Read Mass Flow Rate"=w819:bool, "error out"=w828:errorcluster)  [unwired: 2 out]
                  n454 = Equal To 0?(x=w821) -> (x = 0?=w822:bool)
                  n455 = Wait (ms)(milliseconds to wait=w830) -> ()  [unwired: 1 out]
                  n456 = local read "Stop Test Seqence"() -> (w818:bool)
                  n457 = Unbundle(w826) -> ("UE"=w835:bool, "LE"=w834:bool, "COMP"=w833:bool)  [unwired: 1 out]
                  n458 = local write "Log Data"(w827) -> ()
                  n459 = local write "POWER"(w826) -> ()
                  n460 = Compound Arithmetic op=OR(w835, w834, w833, w818) -> (w820:bool)
                  n461 = Or(x=w822, y=w820) -> (x .or. y?=w823:bool)
                  n462 = case shown="True" w823 {
                    tunnel: w827 -> [_ w836]
                    frame False {
                    }
                    frame True {
                      n463 = Index Array(array=w836, index (row)=1) -> (element=w837:string[])  [unwired: 1 in]
                      n464 = local read "FileName"() -> (w839:path)
                      n465 = call-poly <vilib>:"Write To Spreadsheet File.vi"("delimiter (\\t)"="," ("delimiter (\\t)"), "append to file? (new file:F)"=TRUE, "1D data"=w837, "file path (dialog if empty)"=w839) -> ()  [unwired: 4 in, 1 out]
                    }
                  }
                  n466 = local write "Voltage"(w819) -> ()
                }
                n467 = local read "GEA2 HyperData"() -> (w761:bool)
                n468 = flat-sequence {
                  tunnel: w772 -> [w799]
                  tunnel: [w798] -> w770
                  frame #0 {
                    n469 = local read "FileName"() -> (w795:path)
                    n470 = call "Log String to Spreadsheet.vi"("String"="Power Off", "error in (no error)"=w799, "FileName"=w795) -> ("error out"=w798:errorcluster)  [unwired: 8 in]
                    n471 = local write "PowerON"(FALSE ("PowerON")) -> ()
                  }
                }
                n472 = local read "Water Heater GEA2 Data"() -> (w762:T1)
                n473 = local read "Chanel List"() -> (w774:string)
                n474 = local read "MW100"() -> (w784:refnum<visa-resource-name>)
                n475 = control-ref of="Tank Display"() -> (w791:refnum<vi>)
                n476 = local read "Use Agilent?"() -> (w765:bool)
                n477 = local read "Label Array"() -> (w764:string[])
                n478 = call "Delay mS.vi"("Error In"=w770, "milliseconds to wait"=w769) -> ("Error Out"=w771:errorcluster)  [unwired: 13 in]
                n479 = call "Generic - DO1.vi"("VISA session"=w784, 2:w792, "Channel_Enum"=w789, "Relay Status (0:CLOSED)"=enum8{"CLOSED", "OPEN"}."CLOSED", "Error In"=w771) -> ("error out"=w773:errorcluster)  [unwired: 9 in, 1 out]
                n480 = local read "Calibration File Array"() -> (w763:dbl[][])
                n481 = local read "Equipment"() -> (w790:T5)
                n482 = call "Gather Test Data - Heatup Test new.vi"("Power Analyzer"=w774, "GEA2?"=w792, "Equipment"=w790, "WT210 Current"=w761, "Tank Display Ref"=w791, "MW100 TC Headers"=w765, 9:"Calibration Coefficients"=w763, "error in (no error)"=w773, 13:"Calibration Coefficients"=w762, 14:w764) -> ("Output Data"=w778:string[][], "POWER"=w776:T8, "Read Mass Flow Rate"=w767:bool, "error out"=w781:errorcluster)  [unwired: 2 out]
                n483 = local write "Voltage"(w767) -> ()
                n484 = Index Array(array=w778, index (row)=1) -> (element=w777:string[])  [unwired: 1 in]
                n485 = local write "POWER"(w776) -> ()
                n486 = local read "FileName"() -> (w787:path)
                n487 = local write "Log Data"(w778) -> ()
                n488 = call-poly <vilib>:"Write To Spreadsheet File.vi"("delimiter (\\t)"="," ("delimiter (\\t)"), "append to file? (new file:F)"=TRUE, "1D data"=w777, "file path (dialog if empty)"=w787) -> ()  [unwired: 4 in, 1 out]
              }
            }
          }
          frame True {
            (unwired) string[] ["Init Draw", "Draw", "Term Draw", "Wait for Cutout", "Wait for Temp Decl", "Wait for Purge", "Purge", "Wait for Next Draw"]  # First Draw States SE
            # "3 cases.  First Draw, Need Max temp.\nIntermediate draws don't and might not cutoff.\nLast draw won't wait for a purge condition and need\nmax temp."
            n489 = while {
              shift-right: [w873] -> w846
              shift-left: w842 -> [w866]
              tunnel: [w862] -> _
              i -> [w870]
              stop <- w863 stop-if-true
              n490 = local read "DrawCount"() -> (w864:i32)
              n491 = Number To Decimal String(number=w870) -> (decimal integer string=w856:string)  [unwired: 1 in]
              n492 = local read "Dispense Times"() -> (w865:dbl[])
              n493 = local read "t*=0"() -> (w859:dbl)
              n494 = call "E-Time.vi"("error in (no error)"=w866) -> ("error out"=w873:errorcluster, "Elapsed Time (sec)"=w868:dbl)  [unwired: 8 in, 1 out]
              n495 = Index Array(array=w865, index=w864) -> (element=w860:dbl)
              n496 = Add(x=w859, y=w860) -> (x+y=w854:dbl)
              n497 = Subtract(x=w868, y=w859) -> (x-y=w869:dbl)
              n498 = Unbundle By Name(w866) -> ("status"=w861:bool)
              n499 = local read "Stop Test Seqence"() -> (w853:bool)
              n500 = Number To Fractional String(number=w854) -> (F-format string=w858:string)  [unwired: 3 in]
              n501 = Greater Or Equal?(x=w869, y=w860) -> (x >= y?=w862:bool)
              n502 = local read "T1"() -> (w867:u32)
              n503 = Concatenate Strings("WAIT FOR T=" ("String"), w858, ".  ", w856, " checks." ("string")) -> (w872:string)
              n504 = call "String_in_Reference.vi"("String"=w872) -> ()  [unwired: 18 in, 1 out]
              n505 = Compound Arithmetic op=OR(w862, w861, w853) -> (w863:bool)
              n506 = Wait (ms)(milliseconds to wait=w867) -> ()  [unwired: 1 out]
            }
            n507 = flat-sequence {
              tunnel: [w851] -> w847
              tunnel: w846 -> [w851]
              tunnel: [w850] -> w843
              frame #0 {
                n508 = local read "DrawCount"() -> (w852:i32)
                n509 = Increment(x=w852) -> (x+1=w850:i32)
                n510 = local write "DrawCount"(w850) -> ()
              }
            }
            n511 = Equal?(x=w843, y=w844) -> (x = y?=w845:bool)
            n512 = case shown="True" w845 {
              tunnel: [w878 w881] -> w849
              tunnel: [w877 w882] -> w848
              tunnel: w847 -> [w877 w882]
              tunnel: w843 -> [w875 _]
              frame False {
                n513 = Equal?(x=w875, y=1) -> (x = y?=w876:bool)
                n514 = case shown="True" w876 {
                  tunnel: [w879 w880] -> w878
                  frame False {
                    w879 = string[] ["Init Draw", "Draw", "Term Draw", "Wait for Purge", "Purge", "Wait for Next Draw"]  # Draw States
                    # "Intermediate Draws"
                  }
                  frame True {
                    w880 = string[] ["Init Draw", "Draw", "Term Draw", "Wait for Purge", "Purge", "Wait for Next Draw"]  # First Draw States
                    # "First Draw"
                  }
                }
              }
              frame True {
                w881 = string[] ["Init Draw", "Draw", "Term Draw", "Wait for Cutout", "Wait for Temp Decl", "Wait for Next Draw"]  # Last Draw States
                w883 = TRUE ("Special Last Draw")
                # "Last Draws"
                n515 = local write "Special Last Draw"(w883) -> ()
                "LastDraw" <- w883
              }
            }
          }
        }
      }
      frame "Draw" {
        n516 = flat-sequence {
          tunnel: [w903] -> w889
          tunnel: w888 -> [w903]
          frame #0 {
            "Drawing" <- TRUE
          }
        }
        n517 = while {
          shift-right: [w914] -> w885
          shift-left: w889 -> [w938]
          tunnel: w895 -> [w929]
          tunnel: [w929] -> w891
          shift-right: [w948] -> _
          shift-left: 15.0 ("GPM") -> [w947]
          shift-right: [w934] -> _
          shift-left: 0.0 ("GPM") -> [w935]
          tunnel: w890 -> [_]
          stop <- w950 stop-if-true
          # "T*max is max outlet temp."
          # "Sum of Temperatures"
          # "time to read"
          # "Start Special Case Immediately.  If after 30 sec, T< last\ntime, stop and discard measuremnts."
          # "(For Last Draw, If after 30 sec, T< last tmin, stop and discard measurements, else continue)"
          # "Record output water temp after 15 secs, and at 5 sec intervals thereafter\nMonitor inlet water temp, must be 58 +/- 2 F\nTerminate draw when output temp = T*max -25F, record T*min"
          n518 = local read "Current Draw Start Time"() -> (w945:dbl)
          n519 = local read "Label Array"() -> (w933:string[])
          n520 = call "E-Time.vi"("error in (no error)"=w938) -> ("error out"=w931:errorcluster, "Elapsed Time (sec)"=w911:dbl)  [unwired: 8 in, 1 out]
          n521 = stacked-sequence {
            seq-local: [w954 _ _ _ _] -> [_ w968 w972 w980 w986]
            tunnel: [_ w970 _ _ _] -> w915
            tunnel: w931 -> [w964 _ _ _ _]
            tunnel: [_ _ w973 _ _] -> w926
            tunnel: [w963 _ _ _ _] -> w930
            tunnel: w929 -> [w960 _ _ _ _]
            tunnel: [_ _ _ _ w984] -> w912
            tunnel: [_ w967 _ _ _] -> w917
            tunnel: w933 -> [w955 _ _ _ _]
            tunnel: [w954 _ _ _ _] -> w932
            tunnel: w911 -> [_ w966 _ w976 _]
            frame #0 {
              n522 = local read "Calibration File Array"() -> (w953:dbl[][])
              n523 = local read "Water Heater GEA2 Data"() -> (w952:T1)
              n524 = local read "GEA2 HyperData"() -> (w951:bool)
              n525 = local read "Equipment"() -> (w957:T5)
              n526 = control-ref of="Tank Display"() -> (w959:refnum<vi>)
              n527 = local read "Chanel List"() -> (w961:string)
              n528 = call "Gather Test Data - Heatup Test new.vi"("Power Analyzer"=w961, "GEA2?"=w960, "Equipment"=w957, "WT210 Current"=w951, "Tank Display Ref"=w959, "MW100 TC Headers"=FALSE ("Agilent?"), 9:"Calibration Coefficients"=w953, "error in (no error)"=w964, 13:"Calibration Coefficients"=w952, 14:w955) -> ("Output Data"=w954:string[][], "POWER"=w962:T8, "Read Mass Flow Rate"=w958:bool, "error out"=w963:errorcluster)  [unwired: 2 out]
              n529 = local write "POWER"(w962) -> ()
              n530 = local write "Voltage"(w958) -> ()
            }
            frame #1 {
              # "Tmin assumed to\nbe last TOUT"
              n531 = local write "Log Data"(w968) -> ()
              n532 = call "Array_Search_For_Num.vi"("N Rows of Data"=w968, "Title?"="FLOW(GPM)" ("String")) -> ("number"=w967:dbl)  [unwired: 12 in, 1 out]
              n533 = call "Chart - Buffer Data.vi"("Time"=w966, "Data"=w967) -> ("XY chart data"=→"Flowmeter":cluster{"x":dbl, "y":dbl}[])  [unwired: 9 in]
              n534 = local read "Tank Display"() -> (w971:T9)
              n535 = Unbundle By Name(w971) -> ("TOUT"=w970:dbl)
            }
            frame #2 {
              n536 = call "Array_Search_For_Num.vi"("N Rows of Data"=w972, "Title?"="GALLONS") -> ("number"=w973:dbl)  [unwired: 12 in, 1 out]
            }
            frame #3 {
              n537 = local read "T*min"() -> (w978:dbl)
              n538 = call "Array_Search_For_Num.vi"("N Rows of Data"=w980, "Title?"="RTD_OUT" ("String")) -> ("number"=w977:dbl)  [unwired: 12 in, 1 out]
              n539 = local read "T*Max"() -> (w981:dbl)
              n540 = Max & Min(x=w981, y=w977) -> (max(x,y)=w982:dbl)  [unwired: 1 out]
              n541 = call "Chart - Buffer Data.vi"("Time"=w976, "Data"=w977) -> ("XY chart data"=→"RTD Out":cluster{"x":dbl, "y":dbl}[])  [unwired: 9 in]
              n542 = Max & Min(x=w977, y=w978) -> (min(x,y)=w979:dbl)  [unwired: 1 out]
              n543 = local write "T*Max"(w982) -> ()
              n544 = local write "T*min"(w979) -> ()
            }
            frame #4 {
              n545 = call "Array_Search_For_Num.vi"("N Rows of Data"=w986, "Title?"="Tc_down" ("String")) -> ("number"=w984:dbl)  [unwired: 12 in, 1 out]
              "TcDown" <- w984
            }
          }
          n546 = Subtract(x=w911, y=w945) -> (x-y=w921:dbl)
          n547 = Greater Or Equal?(x=w921, y=w947) -> (x >= y?=w936:bool)
          n548 = case shown="True" w936 {
            tunnel: [w988 w1010] -> w948
            tunnel: w947 -> [w988 w1009]
            tunnel: w930 -> [w989 w993]
            tunnel: [w991 w1008] -> w934
            tunnel: w935 -> [w991 w1007]
            tunnel: [FALSE w1006] -> w946
            tunnel: [w987 w1005] -> w920
            tunnel: [w989 w993] -> w937
            tunnel: w932 -> [_ w995]
            tunnel: w926 -> [_ w994]
            tunnel: w915 -> [_ w992]
            frame False {
              n549 = local read "Gal Target"() -> (w987:dbl)
            }
            frame True {
              n550 = Add(x=5.0, y=w1009) -> (x+y=w1010:dbl)
              "Loop" <- w1010
              n551 = local read "LastDraw"() -> (w1001:bool)
              n552 = Index Array(array=w995, index (row)=1) -> (element=w996:string[])  [unwired: 1 in]
              n553 = local read "FileName"() -> (w998:path)
              n554 = call-poly <vilib>:"Write To Spreadsheet File.vi"("delimiter (\\t)"="," ("delimiter (\\t)"), "append to file? (new file:F)"=TRUE, "1D data"=w996, "file path (dialog if empty)"=w998) -> ()  [unwired: 4 in, 1 out]
              n555 = case shown="False" w1001 {
                tunnel: w994 -> [_ w1019]
                tunnel: w994 -> [w1016 _]
                tunnel: [w1015 w1021] -> w1006
                tunnel: [w1012 w1018] -> w1005
                frame False {
                  n556 = local read "Dispense Schedule"() -> (w1017:dbl[])
                  "Dispense Schedule 2" <- w1017
                  n557 = local read "DrawCount"() -> (w1014:i32)
                  "DrawCount 2" <- w1014
                  n558 = Delete From Array(array=w1017, length=w1014, index=0) -> (deleted portion=w1011:dbl[])  [unwired: 1 out]
                  "deleted portion" <- w1011
                  n559 = Add Array Elements(numeric array=w1011) -> (sum=w1012:dbl)
                  n560 = Greater Or Equal?(x=w1016, y=w1012) -> (x >= y?=w1015:bool)
                }
                frame True {
                  n561 = local read "Dispense Schedule"() -> (w1022:dbl[])
                  n562 = Add Array Elements(numeric array=w1022) -> (sum=w1020:dbl)
                  n563 = Greater Or Equal?(x=w1019, y=w1020) -> (x >= y?=w1021:bool)
                  n564 = Subtract(x=w1020, y=w1019) -> (x-y=w1018:dbl)
                }
              }
              n565 = expression code="x/5-3"(w1010) -> (w1003:dbl)
              n566 = Add(x=w1007, y=w992) -> (x+y=w1008:dbl)
              n567 = Divide(x=w1008, y=w1003) -> (x/y=→"T*Ave":dbl)
              "Volume(Gal.)" <- w994
            }
          }
          "Gal Target" <- w920
          n568 = To Long Integer(number=w920) -> (32bit integer=w916:i32)
          n569 = local read "TempAdj"() -> (w913:dbl)
          n570 = Number To Decimal String(number=w916) -> (decimal integer string=w942:string)  [unwired: 1 in]
          n571 = local read "MW100"() -> (w928:refnum<visa-resource-name>)
          n572 = Concatenate Strings("Draw until " ("string"), w942, "gallons." ("string")) -> (w940:string)
          n573 = call "String_in_Reference.vi"("String"=w940) -> ()  [unwired: 18 in, 1 out]
          n574 = local read "DrawCount"() -> (w905:i32)
          n575 = local read "Temperature Schedule"() -> (w909:dbl[])
          n576 = local read "Flow Rate Schedule"() -> (w910:dbl[])
          n577 = Decrement(x=w905) -> (x-1=w906:i32)
          n578 = local read "Stop Test Seqence"() -> (w939:bool)
          n579 = Index Array(array=w909, index=w906) -> (element=w907:dbl)
          n580 = Subtract(x=w907, y="RTDin to Downspout Offset") -> (x-y=w918:dbl)
          n581 = Index Array(array=w910, index=w906) -> (element=w908:dbl)
          n582 = call "HEWH Flow and Temp Adjustment.vi"("MW100"=w928, "FlowReading"=w917, "Flow In"="Flow Adj", "K(0.1)"="K(0.1)", "TempReading"=w912, "Error In"=w937, "FlowTarget"=w908, "Temp Target"=w918, "Temp In"=w913, "Semiphore"=w929, "Elapsed Time (sec)"=w921, "Flow Adjust Time (3s)"="Adj Time") -> ("Flow Out"=w923:dbl, "Temp Out"=w925:dbl, "Error Out"=w914:errorcluster)  [unwired: 5 in]
          n583 = Unbundle By Name(w914) -> ("status"=w949:bool)
          n584 = local write "TempAdj"(w925) -> ()
          n585 = local write "Flow Adj"(w923) -> ()
          n586 = local read "T5"() -> (w944:u32)
          n587 = Compound Arithmetic op=OR(w949, w946, w939) -> (w950:bool)
          n588 = Wait (ms)(milliseconds to wait=w944) -> ()  [unwired: 1 out]
        }
        n589 = case shown="No Error" w885 {
          selector: w885 -> [w896 w902]
          tunnel: [w898 string[] ["Finish"] ("States")] -> w886
          tunnel: w887 -> [w898 _]
          tunnel: [w897 w902] -> w884
          frame No Error {
            n590 = flat-sequence {
              tunnel: [w900] -> w897
              tunnel: w896 -> [w900]
              frame #0 {
                n591 = local write "Drawing"(FALSE) -> ()
              }
            }
          }
          frame Error {
          }
        }
      }
      frame "Draw0" {
        n592 = local read "Flow Adj"() -> (w1023:dbl)
        n593 = while {
          shift-right: [w1058] -> w1029
          shift-left: w1026 -> [w1059]
          shift-right: [w1061] -> _
          shift-left: w1023 -> [w1065]
          tunnel: w1030 -> [w1060]
          tunnel: [w1060] -> w1025
          tunnel: w1024 -> [_]
          stop <- w1066 stop-if-true
          # "Draw until power for heating kicks on."
          n594 = call "E-Time.vi"("error in (no error)"=w1059) -> ("error out"=w1063:errorcluster, "Elapsed Time (sec)"=w1036:dbl)  [unwired: 8 in, 1 out]
          n595 = local read "Label Array"() -> (w1042:string[])
          n596 = stacked-sequence {
            seq-local: [w1091 _ _ _] -> [_ w1102 w1107 w1111]
            tunnel: w1063 -> [w1093 _ _ _]
            tunnel: [w1092 _ _ _] -> w1051
            tunnel: w1060 -> [w1089 _ _ _]
            tunnel: [_ _ _ w1109] -> w1044
            tunnel: [_ w1100 _ _] -> w1043
            tunnel: w1042 -> [w1084 _ _ _]
            tunnel: [w1083 _ _ _] -> w1037
            tunnel: w1036 -> [_ w1099 w1104 _]
            frame #0 {
              n597 = local read "Water Heater GEA2 Data"() -> (w1081:T1)
              n598 = local read "GEA2 HyperData"() -> (w1080:bool)
              n599 = local read "Equipment"() -> (w1086:T5)
              n600 = control-ref of="Tank Display"() -> (w1088:refnum<vi>)
              n601 = local read "Chanel List"() -> (w1090:string)
              n602 = local read "Calibration File Array"() -> (w1082:dbl[][])
              n603 = call "Gather Test Data - Heatup Test new.vi"("Power Analyzer"=w1090, "GEA2?"=w1089, "Equipment"=w1086, "WT210 Current"=w1080, "Tank Display Ref"=w1088, "MW100 TC Headers"=FALSE ("Agilent?"), 9:"Calibration Coefficients"=w1082, "error in (no error)"=w1093, 13:"Calibration Coefficients"=w1081, 14:w1084) -> ("Output Data"=w1091:string[][], "POWER"=w1083:T8, "Read Mass Flow Rate"=w1087:bool, "error out"=w1092:errorcluster)  [unwired: 2 out]
              n604 = local write "POWER"(w1083) -> ()
              n605 = local write "Voltage"(w1087) -> ()
              n606 = local read "FileName"() -> (w1096:path)
              n607 = Index Array(array=w1091, index (row)=1) -> (element=w1098:string[])  [unwired: 1 in]
              n608 = call-poly <vilib>:"Write To Spreadsheet File.vi"("delimiter (\\t)"="," ("delimiter (\\t)"), "append to file? (new file:F)"=TRUE, "1D data"=w1098, "file path (dialog if empty)"=w1096) -> ()  [unwired: 4 in, 1 out]
            }
            frame #1 {
              # "Tmin assumed to\nbe last TOUT"
              n609 = local write "Log Data"(w1102) -> ()
              n610 = call "Array_Search_For_Num.vi"("N Rows of Data"=w1102, "Title?"="FLOW(GPM)" ("String")) -> ("number"=w1100:dbl)  [unwired: 12 in, 1 out]
              n611 = call "Chart - Buffer Data.vi"("Time"=w1099, "Data"=w1100) -> ("XY chart data"=→"FlowMeter During Draw0":cluster{"x":dbl, "y":dbl}[])  [unwired: 9 in]
            }
            frame #2 {
              n612 = call "Array_Search_For_Num.vi"("N Rows of Data"=w1107, "Title?"="RTD_OUT" ("String")) -> ("number"=w1105:dbl)  [unwired: 12 in, 1 out]
              n613 = call "Chart - Buffer Data.vi"("Time"=w1104, "Data"=w1105) -> ("XY chart data"=→"RTD Out 0":cluster{"x":dbl, "y":dbl}[])  [unwired: 9 in]
            }
            frame #3 {
              n614 = call "Array_Search_For_Num.vi"("N Rows of Data"=w1111, "Title?"="Tc_down" ("String")) -> ("number"=w1109:dbl)  [unwired: 12 in, 1 out]
              "TcDown 0" <- w1109
            }
          }
          n615 = local read "RTDin to Downspout Offset"() -> (w1041:dbl)
          n616 = local read "Adj Time"() -> (w1039:dbl)
          n617 = local read "K(0.1)"() -> (w1040:dbl)
          n618 = local read "TempAdj"() -> (w1046:dbl)
          n619 = local read "MW100"() -> (w1048:refnum<visa-resource-name>)
          n620 = local read "Temperature Schedule"() -> (w1035:dbl[])
          n621 = local read "Flow Rate Schedule"() -> (w1034:dbl[])
          n622 = local read "DrawCount"() -> (w1033:i32)
          n623 = call "String_in_Reference.vi"("String"="Draw until heating turns on." ("string")) -> ()  [unwired: 18 in, 1 out]
          n624 = Index Array(array=w1034, index=w1033) -> (element=w1032:dbl)
          n625 = Index Array(array=w1035, index=w1033) -> (element=w1031:dbl)
          n626 = Subtract(x=w1031, y=w1041) -> (x-y=w1047:dbl)
          n627 = call "HEWH Temp Adjustment.vi"("VISA session"=w1048, 2:w1060, "Degrees Target"=w1047, "Degrees reading"=w1044, "New Temp Reading \nfrom last adjustment"=w1046, "Error In"=w1051, 12:w1036, 13:w1039, "K(0.1)"=w1040) -> ("VISA session out"=w1049:refnum<visa-resource-name>, "Degree setting Out"=w1045:dbl, "Error Out"=w1050:errorcluster)  [unwired: 4 in]
          n628 = local write "TempAdj"(w1045) -> ()
          n629 = call "HEWH Flow Adjustment.vi"("VISA session"=w1049, 2:w1060, "GPM Target(3)"=w1032, "GPM reading"=w1043, "New GPM Reading \nfrom last adjustment"=w1065, "Error In"=w1050, "Output Input (Percent)"=w1036, 13:w1039, "K(0.2)"=w1040) -> ("Flow rate setting Out"=w1061:dbl, "Error Out"=w1058:errorcluster)  [unwired: 3 in, 2 out]
          n630 = local read "Stop Test Seqence"() -> (w1052:bool)
          n631 = disable-structure shown="Enabled" {
            disable-tunnel: [w1071 w1072 w1079 _] -> w1057
            disable-tunnel: [w1070 w1072 w1078 _] -> w1056
            disable-tunnel: [w1069 w1072 w1077 _] -> w1055
            disable-tunnel: [w1068 w1074 w1076 _] -> w1054
            disable-tunnel: w1037 -> [w1067 w1073 w1075 _]
            frame Disabled {
              n632 = Unbundle(w1067) -> ("UE"=w1068:bool, "LE"=w1069:bool, "COMP"=w1070:bool, "FANS"=w1071:bool)
            }
            frame Disabled {
              n633 = Unbundle(w1073) -> ("UE"=w1074:bool, "LE"=w1072:bool)  [unwired: 2 out]
            }
            frame Enabled {
              n634 = Unbundle(w1075) -> ("UE"=w1076:bool, "LE"=w1077:bool, "COMP"=w1078:bool, "FANS"=w1079:bool)
            }
            frame Disabled {
            }
          }
          n635 = Unbundle By Name(w1058) -> ("status"=w1064:bool)
          n636 = local write "Flow Adj"(w1061) -> ()
          n637 = local read "T5"() -> (w1062:u32)
          n638 = Compound Arithmetic op=OR(w1054, w1055, w1056, w1057, w1064, w1052, "Skip Draw0") -> (w1066:bool)
          n639 = Wait (ms)(milliseconds to wait=w1062) -> ()  [unwired: 1 out]
        }
      }
      frame "Term Draw" {
        # "For the Macro, we need Term Draw, and Draw Result in consecutive lines of data.  Thus the \"drawing\" semiphore flag."
        # "Energy(Wh)"
        n640 = flat-sequence {
          tunnel: [w1150] -> w1118
          tunnel: w1117 -> [w1150]
          frame #0 {
            n641 = local write "Drawing"(TRUE ("Drawing")) -> ()
          }
        }
        n642 = local read "Expansion Tank?"() -> (w1123:bool)
        n643 = local read "MW100"() -> (w1120:refnum<visa-resource-name>)
        n644 = call "HEWH Set Valves.vi"("VISA session"=w1120, 2:w1121, "Pressurize Tank?"=w1123, "Valve Bank Setting"=ValveBankPositions."Heating", "Error In"=w1118) -> ("Error Out"=w1122:errorcluster)  [unwired: 9 in, 1 out]
        n645 = local read "Calibration File Array"() -> (w1114:dbl[][])
        n646 = local read "Water Heater GEA2 Data"() -> (w1113:T1)
        n647 = call "HEWH Totalize Flow Control.vi"("VISA session"=w1120, 2:w1121, "Totalize Flow"=FALSE, "error in (no error)"=w1122) -> ("error out"=w1125:errorcluster)  [unwired: 10 in, 1 out]
        n648 = local read "Use Agilent?"() -> (w1128:bool)
        n649 = local read "Chanel List"() -> (w1139:string)
        n650 = local read "Label Array"() -> (w1127:string[])
        n651 = local read "Equipment"() -> (w1131:T5)
        n652 = local read "Semiphore"() -> (w1138:T6)
        n653 = local read "GEA2 HyperData"() -> (w1112:bool)
        n654 = control-ref of="Tank Display"() -> (w1140:refnum<vi>)
        n655 = call "Gather Test Data - Heatup Test new.vi"("Power Analyzer"=w1139, "GEA2?"=w1138, "Equipment"=w1131, "WT210 Current"=w1112, "Tank Display Ref"=w1140, "MW100 TC Headers"=w1128, 9:"Calibration Coefficients"=w1114, "error in (no error)"=w1125, 13:"Calibration Coefficients"=w1113, 14:w1127) -> ("Output Data"=w1129:string[][], "POWER"=w1126:T8, "Read Mass Flow Rate"=w1132:bool, "error out"=w1130:errorcluster)  [unwired: 2 out]
        n656 = local write "Voltage"(w1132) -> ()
        n657 = local write "POWER"(w1126) -> ()
        n658 = local read "Discard Last Draw"() -> (w1141:bool)
        n659 = Index Array(array=w1129, index (row)=1) -> (element=w1135:string[])  [unwired: 1 in]
        n660 = local read "FileName"() -> (w1133:path)
        n661 = call-poly <vilib>:"Write To Spreadsheet File.vi"("delimiter (\\t)"="," ("delimiter (\\t)"), "append to file? (new file:F)"=TRUE, "1D data"=w1135, "file path (dialog if empty)"=w1133) -> ()  [unwired: 4 in, 1 out]
        n662 = case shown="False" w1141 {
          tunnel: [w1168 w1173] -> w1143
          tunnel: w1142 -> [w1167 w1173]
          tunnel: [w1160 w1172] -> w1116
          tunnel: w1130 -> [w1151 w1172]
          tunnel: w1121 -> [_ _]
          tunnel: w1129 -> [w1154 _]
          frame False {
            n663 = local read "Total Gallons Drawn"() -> (w1157:dbl)
            n664 = local read "Volume(Gal.)"() -> (w1156:dbl)
            n665 = call "Array_Search_For_Num.vi"("N Rows of Data"=w1154, "Title?"="Energy(Wh)") -> ("number"=w1152:dbl)  [unwired: 12 in, 1 out]
            "WattHours" <- w1152
            n666 = local read "T*Ave"() -> (w1170:dbl)
            n667 = local read "T*Max"() -> (w1169:dbl)
            n668 = local read "T*min"() -> (w1171:dbl)
            n669 = call "E-Time.vi"("error in (no error)"=w1151) -> ("error out"=w1160:errorcluster, "Elapsed Time (sec)"=w1161:dbl)  [unwired: 8 in, 1 out]
            n670 = Add(x=w1156, y=w1157) -> (x+y=→"Total Gallons Drawn":dbl)
            n671 = Build Array(w1161, w1171, w1170, w1169, w1156, w1152) -> (w1166:dbl[])
            n672 = Build Array (concatenate)(w1167, w1166) -> (w1168:dbl[][])
            n673 = Number To Fractional String(number=w1166) -> (F-format string=w1164:string[])  [unwired: 3 in]
            n674 = local read "FileName"() -> (w1159:path)
            n675 = Build Array (concatenate)("Draw Result(time;T*min;T*ave;T*max; Volume(Gal. for M*);WattHours)", w1164) -> (w1163:string[])
            n676 = call-poly <vilib>:"Write To Spreadsheet File.vi"("delimiter (\\t)"="," ("delimiter (\\t)"), "append to file? (new file:F)"=TRUE, "1D data"=w1163, "file path (dialog if empty)"=w1159) -> ()  [unwired: 4 in, 1 out]
          }
          frame True {
          }
        }
        n677 = flat-sequence {
          tunnel: [w1148] -> w1115
          tunnel: w1116 -> [w1148]
          frame #0 {
            n678 = local write "Drawing"(FALSE ("Drawing")) -> ()
          }
        }
        n679 = case shown="Error" w1115 {
          selector: w1115 -> [w1174 w1177]
          tunnel: [w1175 string[] ["Finish"] ("States")] -> w1145
          tunnel: w1146 -> [w1175 _]
          tunnel: [w1174 w1177] -> w1144
          frame No Error {
          }
          frame Error {
          }
        }
      }
      frame "Finish", Default {
        n680 = local write "Status Tabl"(8 ("index")) -> ()
        n681 = case shown="No Error" w1181 {
          selector: w1181 -> [w1199 w1216]
          tunnel: [w1205 w1219] -> w1194
          tunnel: w1193 -> [w1205 w1219]
          tunnel: [w1200 errorcluster {"status"=FALSE, "code"=0, "source"=""} ("error IO")] -> w1183
          tunnel: w1179 -> [w1201 _]
          frame No Error {
            n682 = Equal?(x=w1201, y="Finish") -> (x = y?=w1204:bool)
            n683 = Concatenate Strings("False State: " ("string"), w1201) -> (w1198:string)
            n684 = case shown="True" w1204 {
              tunnel: [w1206 w1209] -> w1200
              tunnel: w1199 -> [w1206 w1208]
              tunnel: w1198 -> [_ w1207]
              frame True {
              }
              frame False {
                n685 = Bundle(cluster=w1208, "source"=w1207) -> (w1209:errorcluster)  [unwired: 2 in]
              }
            }
          }
          frame Error {
            n686 = Unbundle(w1216) -> ("code"=w1214:i32, "source"=w1211:string)  [unwired: 1 out]
            n687 = Number To Exponential String(number=w1214) -> (E-format string=w1213:string)  [unwired: 3 in]
            n688 = Concatenate Strings("ERROR: ", w1213, ": " ("string"), w1211) -> (w1210:string)
            n689 = local read "FileName"() -> (w1217:path)
            n690 = call "Log String to Spreadsheet.vi"("String"=w1210, "FileName"=w1217) -> ()  [unwired: 9 in, 1 out]
          }
        }
        n691 = Unbundle By Name(w1192) -> ("MW100"=w1184:refnum<visa-resource-name>)
        n692 = call "YKMW100 Get Error Log.vi"("VISA session"=w1184, 2:w1178, "error in (no error)"=w1183) -> ("dup VISA session"=w1188:refnum<visa-resource-name>, "Error History"=→"Error History":string[], "error out"=w1189:errorcluster)  [unwired: 9 in, 1 out]
        n693 = call "YKMW100 Get Com Log.vi"("VISA session"=w1188, "Semiphore"=w1178, "error in (no error)"=w1189) -> ("Com History"=→"Com History":string[], "error out"=w1185:errorcluster)  [unwired: 9 in, 2 out]
        n694 = flat-sequence {
          tunnel: w1185 -> [w1196]
          tunnel: [w1196] -> w1182
          tunnel: w1182 -> [_]
          tunnel: w1181 -> [w1197]
          tunnel: [w1197] -> w1180
          frame #0 {
            w1195 = TRUE ("Stop Logging")
            n695 = local write "Stop Logging"(w1195) -> ()
            n696 = property on="Stop Logging" class="Bool (strict)"("Val(Sgnl)"=w1195) -> ()  [unwired: 2 in, 2 out]
          }
          frame #1 {
          }
        }
      }
    }
    n697 = Build Array (concatenate)(w41, w33) -> (w40:string[])
    "Executaion Sequence" <- w40
    n698 = Equal?(x=w33, y="Finish") -> (x = y?=w50:bool)
    n699 = local read "T2"() -> (w42:u32)
    n700 = Wait Until Next ms Multiple(millisecond multiple=w42) -> ()  [unwired: 1 out]
  }
  "Error Out" <- w17
  "Test Data" <- w14
  n701 = event shown="[1] \"Init Complete\", \"Stop Logging\": Value Change" {
    selector: _ -> [_ _]
    dyn-events: _ -> [_ _]
    timeout: _ -> [_ _]
    event Timeout {
      n702 = event-data() -> ()  [unwired: 1 in, 2 out]
    }
    event "Init Complete", "Stop Logging": Value Change {
      w1221 = u8 13 items=["RQST_SOFTWARE_VERSION", "RQST_T2_RESISTANCE", "RQST_T3A_RESISTANCE", "RQST_T3B_RESISTANCE", "RQST_T4_RESISTANCE", "RQST_T5_RESISTANCE", "RQST_IDLB_RESISTANCE", "RQST_MODE_SELECT_RESISTANCE", "RQST_DATA_FROM_MEMORY", "RQST_DATA_FROM_DATA_FLASH", "RQST_SS_FAULT_COUNTS", "RQST_OTHER_FAULT_COUNTS", "CMD_CLEAR_FAULT_COUNTS", "RQST_HYPERTERM_OUTPUT_DATA", "CMD_RESET_FILTER_TIMES", "CMD_WRITE_SETPOINTS", "CMD_TURN_ON_OFF_DLB", "CMD_ENTER_EXIT_FCT_MODE", "CMD_SET_LEDS", "CMD_SET_EEV_DRIVE_LINES", "REQ_READ_KEY_STATUS", "RQST_READ_PERSONALITY", "CMD_ENTER_FACT_MODE", "CMD_RESET", "CMD_RESTORE_EEPROM_DEFAULTS", "CMD_SET_MODEL_NUMBER", "CMD_SET_SERIAL_NUMBER", "RQST_MODEL_NUMBER", "RQST_SERIAL_NUMBER", "CMD_TOGGLE_SERVICE_MODE", "CMD_TOGGLE_UE_SERV", "CMD_TOGGLE_LE_SERV", "CMD_REFRESH_SERVICE_TIMEOUTS", "RQST_DSM_OVERRIDE_STATUS", "RQST_STATUS_QUERY", "RQST_HEM_KWH_DATA", "RQST_SERVICE_ERROR_CODES", "RQST_OVERRIDE_STATUS", "CMD_UPDATE_DSM_LEVEL", "CMD_OVERRIDE_STATUS_CHANGED", "CMD_CLEAR_OVERRIDE_STATUS", "CMD_CLEAR_ENERGY_USAGE_CTRS", "CMD_DSM_OVERRIDES", "CMD_UPDATE_MODE", "CMD_SET_PID_P_DENOMINATOR", "CMD_SET_PID_I_DENOM_UNDER_THR", "CMD_SET_PID_I_DENOM_OVER_THR", "CMD_SET_START_POS_UNDER_THR", "CMD_SET_START_POS_OVER_THR", "CMD_SET_EEV_STOP_POSITION", "CMD_SET_AMBIENT_THRESH_1", "CMD_SET_AMBIENT_THRESH_2", "CMD_SET_AMBIENT_THRESH_3", "CMD_SET_PID_LOW_SH_TARGET", "CMD_SET_PID_MID_SH_TARGET", "RQST_PID_PARAMETERS", "CMD_COMP_OFF", "CMD_TOGGLE_FAN", "CMD_RQST_LED_STATUS", "CMD_UE_2_SECONDS", "CMD_LE_2_SECONDS", "CMD_COMP_ON", "CMD_HP_RUN_6MIN", "RQST_TEMP_RANGE", "RQST_VACATION_RANGE", "RQST_STD_ELEC_RANGE", "RQST_WATER_CAPACITY", "CMD_CANCEL_EEV_POSITION", "CMD_EEV_POSITION", "CMD_SET_CURRENTS", "RQST_SUPPORTED_MODES"] ("Command")
      n703 = event-data() -> ()  [unwired: 1 in, 5 out]
      n704 = call "HEWH_DSM_CMD.vi"("GEA2 Commands and Requests"=w1221) -> ("Input Data"=w1220:T25)  [unwired: 8 in, 1 out]
      n705 = Unbundle By Name(w1220) -> ("Source"=w1226:u8)
      n706 = call "GEA2 Initialize.vi"("Board Index"=0, "Source Address"=w1226) -> ("GEA2 Reference Out"=w1225:refnum<k24>, "error out"=w1224:errorcluster)  [unwired: 11 in, 1 out]
      n707 = while {
        tunnel: [w1237] -> w1228
        shift-right: [w1233] -> w1222
        shift-left: w1224 -> [w1234]
        shift-right: [w1232] -> w1223
        shift-left: w1225 -> [w1235]
        tunnel: w1221 -> [w1231]
        tunnel: w1220 -> [w1230]
        stop <- w1237 stop-if-true
        n708 = local read "Init Complete"() -> (w1236:bool)
        n709 = Wait Until Next ms Multiple(millisecond multiple=u32 1000 ("milliseconds to wait")) -> ()  [unwired: 1 out]
        n710 = case shown="True" w1236 {
          tunnel: w1235 -> [w1238 w1246]
          tunnel: w1234 -> [w1239 w1244]
          tunnel: [w1239 w1243] -> w1233
          tunnel: [w1238 w1242] -> w1232
          tunnel: w1231 -> [_ w1241]
          tunnel: w1230 -> [_ w1240]
          frame False {
          }
          frame True {
            n711 = call "GEA2 Send and Receive Message.vi"("GEA2 Reference In"=w1246, "Input Data"=w1240, "Error In"=w1244) -> ("GEA2 Reference Out"=w1242:refnum<k24>, "Converted Data Out"=w1245:T26, "Error Out"=w1243:errorcluster)  [unwired: 9 in, 1 out]
            n712 = call "GEA2 Message Decoder.vi"("GEA2 Commands and Requests"=w1241, "Coverted Data Out"=w1245) -> ("Water Heater GEA2 Data"=→"Water Heater GEA2 Data":T1)  [unwired: 9 in]
          }
        }
        n713 = local read "Stop Logging"() -> (w1237:bool)
      }
      "StopSerial" <- w1228
      n714 = property on="StopSerial" class="Bool (strict)"("Val(Sgnl)"=w1228) -> ()  [unwired: 2 in, 2 out]
      n715 = call "GEA2 Stop.vi"("GEA2 Reference In"=w1223, "Error In"=w1222) -> ()  [unwired: 13 in, 1 out]
    }
  }
  n716 = while {
    shift-right: [w1256] -> w12
    shift-left: 0 ("milliseconds to wait") -> [w1257]
    shift-right: [w1254] -> _
    shift-left: 0.0 -> [w1250]
    stop <- "Stop Logging" stop-if-true
    # "continuous data gathering"
    n717 = local read "Init Complete"() -> (w1258:bool)
    n718 = Multiply(x="Sample Per.(s)", y=1000.0) -> (x*y=w1251:dbl)
    n719 = local read "T2"() -> (w1249:u32)
    n720 = case shown="True" w1258 {
      tunnel: w1257 -> [w1263 w1275]
      tunnel: [w1263 w1274] -> w1256
      tunnel: [w1262 w1273] -> w1255
      tunnel: w1251 -> [_ w1270]
      tunnel: w1250 -> [_ w1267]
      frame False {
        (unwired) FALSE ("status")
        n721 = call "E-Time.vi"() -> ("Elapsed Time (sec)"=w1262:dbl)  [unwired: 9 in, 2 out]
      }
      frame True {
        n722 = To Long Integer(number=w1270) -> (32bit integer=w1265:i32)
        n723 = Multiply(x=w1267, y=1000.0) -> (x*y=w1269:dbl)
        n724 = To Long Integer(number=w1269) -> (32bit integer=w1266:i32)
        n725 = Subtract(x=w1265, y=w1266) -> (x-y=w1264:i32)
        n726 = In Range and Coerce(upper limit=w1265, x=w1264, lower limit=0) -> (coerced(x)=w1272:i32)  [unwired: 1 out]
        n727 = event shown="[0] Timeout" {
          selector: _ -> [_]
          dyn-events: _ -> [_]
          timeout: w1272 -> [_]
          tunnel: w1275 -> [w1283]
          tunnel: [w1280] -> w1274
          tunnel: [w1279] -> w1273
          event Timeout {
            # "Power Assumed to be on"
            n728 = event-data() -> ()  [unwired: 1 in, 2 out]
            n729 = local read "Calibration File Array"() -> (w1277:dbl[][])
            n730 = flat-sequence {
              tunnel: [w1321] -> w1282
              tunnel: [w1323] -> w1281
              tunnel: [w1322] -> w1279
              frame #0 {
                n731 = local read "Water Heater GEA2 Data"() -> (w1321:T1)
                n732 = local read "Label Array"() -> (w1323:string[])
                n733 = call "E-Time.vi"() -> ("Elapsed Time (sec)"=w1322:dbl)  [unwired: 9 in, 2 out]
              }
            }
            n734 = local read "GEA2 HyperData"() -> (w1276:bool)
            n735 = local read "Use Agilent?"() -> (w1311:bool)
            n736 = local read "Chanel List"() -> (w1312:string)
            n737 = local read "Equipment"() -> (w1314:T5)
            n738 = local read "Semiphore"() -> (w1313:T6)
            n739 = control-ref of="Tank Display"() -> (w1310:refnum<vi>)
            n740 = call "Gather Test Data - Heatup Test new.vi"("Power Analyzer"=w1312, "GEA2?"=w1313, "Equipment"=w1314, "WT210 Current"=w1276, "Tank Display Ref"=w1310, "MW100 TC Headers"=w1311, 9:"Calibration Coefficients"=w1277, 13:"Calibration Coefficients"=w1282, 14:w1281) -> ("Tc Tree"=w1301:dbl[], "Output Data"=w1284:string[][], "POWER"=w1278:T8, "PowerData"=w1300:T32, "Read Mass Flow Rate"=→"Voltage":bool, "error out"=→"Error Datalogging":errorcluster)  [unwired: 1 in]
            "Log Data" <- w1284
            n741 = local write "POWER"(w1278) -> ()
            n742 = Array To Cluster(array=w1301) -> (cluster=w1291:T30)
            n743 = Unbundle(w1278) -> ("UE"=w1298:bool, "LE"=w1296:bool, "COMP"=w1297:bool, "FANS"=w1308:bool)
            n744 = Build Array(w1291) -> (→"Temps":T12)
            n745 = Boolean To (0,1)(Boolean=w1308) -> (0, 1=w1309:i16)
            n746 = Unbundle By Name(w1300) -> ("Power (Watts)"=w1302:dbl)
            n747 = Boolean To (0,1)(Boolean=w1298) -> (0, 1=w1303:i16)
            n748 = Boolean To (0,1)(Boolean=w1297) -> (0, 1=w1307:i16)
            n749 = Boolean To (0,1)(Boolean=w1296) -> (0, 1=w1305:i16)
            n750 = Increment(x=w1283) -> (x+1=w1280:i32)
            "Number of Records" <- w1280
            n751 = expression code="2*x"(w1307) -> (w1289:i16)
            n752 = Index Array(array=w1284, index (row)=1) -> (element=w1285:string[])  [unwired: 1 in]
            n753 = expression code="3*x"(w1305) -> (w1306:i16)
            n754 = expression code="4*x"(w1303) -> (w1304:i16)
            n755 = call "Array_Search_For_Num.vi"("N Rows of Data"=w1284, "Title?"="GALLONS") -> ("number"=→"Gallons Chart":dbl)  [unwired: 12 in, 1 out]
            n756 = Build Array(w1302, w1304, w1306, w1289, w1309) -> (w1293:dbl[])
            n757 = Array To Cluster(array=w1293) -> (cluster=w1295:T34)
            n758 = flat-sequence {
              tunnel: w1285 -> [w1316]
              frame #0 {
                # "Dont record during draw"
                n759 = local read "Drawing"() -> (w1315:bool)
                n760 = case shown="False" w1315 {
                  tunnel: w1316 -> [w1319 _]
                  frame False {
                    n761 = local read "FileName"() -> (w1320:path)
                    n762 = call-poly <vilib>:"Write To Spreadsheet File.vi"("delimiter (\\t)"="," ("delimiter (\\t)"), "append to file? (new file:F)"=TRUE, "1D data"=w1319, "file path (dialog if empty)"=w1320) -> ()  [unwired: 4 in, 1 out]
                  }
                  frame True {
                  }
                }
              }
            }
            n763 = Build Array(w1295) -> (→"Watt Chart":T14)
          }
        }
      }
    }
    n764 = Wait Until Next ms Multiple(millisecond multiple=w1249) -> ()  [unwired: 1 out]
    n765 = flat-sequence {
      tunnel: w1255 -> [w1260]
      tunnel: [w1259] -> w1254
      frame #0 {
        n766 = call "E-Time.vi"() -> ("Elapsed Time (sec)"=w1261:dbl)  [unwired: 9 in, 2 out]
        n767 = Subtract(x=w1261, y=w1260) -> (x-y=w1259:dbl)
      }
    }
  }
  n768 = while {
    stop <- w1325 stop-if-true
    n769 = local read "T3"() -> (w1326:u32)
    n770 = To Long Integer(number=w1326) -> (32bit integer=w1324:i32)
    n771 = event shown="[1] \"stop\": Value Change" {
      selector: _ -> [_ _ _ _ _]
      dyn-events: _ -> [_ _ _ _ _]
      timeout: w1324 -> [_ _ _ _ _]
      tunnel: [_ "stop" _ _ _] -> w1325
      event Timeout {
        n772 = event-data() -> ()  [unwired: 1 in, 2 out]
        n773 = call "String_in_Reference.vi"() -> ("String Out"=→"STATUS":string)  [unwired: 19 in]
        n774 = call "E-Time.vi"() -> ("Elapsed Time (sec)"=→"Elapsed.Time (H:M:S)":dbl)  [unwired: 9 in, 2 out]
      }
      event "stop": Value Change {
        n775 = event-data() -> ()  [unwired: 1 in, 5 out]
        n776 = case shown="True" "stop" {
          frame False {
          }
          frame True {
            n777 = stacked-sequence {
              frame #0 {
                w1337 = T33 30 items=["4-20_OUT", "Pres_HI1", "Pres_HI2", "Pres_LOW", "Pres_PIN", "HEATER_TOP", "HEATER_BOT", "T_Shell", "FLOWMETER", "WATT_SENSE", "WH_TICK", "Tc_1", "Tc_2", "Tc_3", "Tc_4", "Tc_5", "Tc_6", "Tc_down", "T_Shell_2", "T_Shell_3", "T_Shell_4", "RTD_IN", "RTD_OUT", "RTD_AMB", "INTF_TEMPFLO", "INTF_READY", "INTF_START", "INTF_STOP", "DRM_LOW", "DRM_HIGH", "PWR_MAIN", "VLV_DUMP", "VLV_OUT", "VLV_IN", "WATT_HOURS", "FLOW(SAMPLE)", "GALLONS", "FLOW(GPM)"] ("Channel_Enum")
                # "Turn off water, and power on, open output valve"
                n778 = local read "Expansion Tank?"() -> (w1333:bool)
                n779 = local read "Semiphore"() -> (w1334:T6)
                n780 = local read "MW100"() -> (w1331:refnum<visa-resource-name>)
                n781 = call "HEWH Set Valves.vi"("VISA session"=w1331, 2:w1334, "Pressurize Tank?"=w1333, "Valve Bank Setting"=ValveBankPositions."Resting") -> ("dup VISA session"=w1335:refnum<visa-resource-name>, "Error Out"=w1336:errorcluster)  [unwired: 10 in]
                n782 = local write "STATUS"("Stopping Test..." ("string")) -> ()
                n783 = call "Generic - DO1.vi"("VISA session"=w1335, 2:w1334, "Channel_Enum"=w1337, "Relay Status (0:CLOSED)"=enum8{"CLOSED", "OPEN"}."OPEN", "Error In"=w1336) -> ()  [unwired: 9 in, 2 out]
              }
              frame #1 {
                n784 = local read "Error Datalogging"() -> (w1340:errorcluster)
                n785 = Unbundle By Name(w1340) -> ("status"=w1339:bool)
                n786 = case shown="True" w1339 {
                  frame False {
                  }
                  frame True {
                    n787 = local read "FileName"() -> (w1341:path)
                    n788 = call "Log String to Spreadsheet.vi"("String"="Error Datalogging", "FileName"=w1341) -> ()  [unwired: 9 in, 1 out]
                  }
                }
              }
              frame #2 {
                n789 = local read "Water Heater GEA2 Data"() -> (w1344:T1)
                n790 = local read "GEA2 HyperData"() -> (w1343:bool)
                n791 = local read "Chanel List"() -> (w1359:string)
                n792 = local read "Equipment"() -> (w1357:T5)
                n793 = local read "Use Agilent?"() -> (w1348:bool)
                n794 = local read "Label Array"() -> (w1347:string[])
                n795 = local read "Semiphore"() -> (w1358:T6)
                n796 = control-ref of="Tank Display"() -> (w1360:refnum<vi>)
                n797 = local read "FileName"() -> (w1350:path)
                n798 = local read "Calibration File Array"() -> (w1345:dbl[][])
                n799 = call "Gather Test Data - Heatup Test new.vi"("Power Analyzer"=w1359, "GEA2?"=w1358, "Equipment"=w1357, "WT210 Current"=w1343, "Tank Display Ref"=w1360, "MW100 TC Headers"=w1348, 9:"Calibration Coefficients"=w1345, 13:"Calibration Coefficients"=w1344, 14:w1347) -> ("Output Data"=w1356:string[][], "POWER"=w1346:T8, "Read Mass Flow Rate"=w1361:bool)  [unwired: 1 in, 3 out]
                n800 = Index Array(array=w1356, index (row)=1) -> (element=w1353:string[])  [unwired: 1 in]
                n801 = local write "POWER"(w1346) -> ()
                n802 = call-poly <vilib>:"Write To Spreadsheet File.vi"("delimiter (\\t)"="," ("delimiter (\\t)"), "append to file? (new file:F)"=TRUE, "1D data"=w1353, "file path (dialog if empty)"=w1350) -> ("new file path (Not A Path if cancelled)"=w1349:path)  [unwired: 4 in]
                n803 = call "Log String to Spreadsheet.vi"("String"="Stopped", "FileName"=w1349) -> ()  [unwired: 9 in, 1 out]
                n804 = local write "Voltage"(w1361) -> ()
              }
              frame #3 {
                n805 = local read "Init Complete"() -> (w1363:bool)
                n806 = local read "Local?"() -> (w1362:bool)
                n807 = And(x=w1362, y=w1363) -> (x .and. y?=w1364:bool)
                n808 = case shown="True" w1364 {
                  tunnel: w1362 -> [_ w1365]
                  frame False {
                  }
                  frame True {
                    n809 = local read "Equipment"() -> (w1367:T5)
                    n810 = call "HEWH CloseEquipmet.vi"("Equipment"=w1367) -> ("Error Out"=w1366:errorcluster)  [unwired: 10 in]
                    n811 = call "Semiphore-Destroy-Local.vi"("Local?"=w1365, "error in (no error)"=w1366) -> ()  [unwired: 17 in, 1 out]
                  }
                }
              }
              frame #4 {
                n812 = local read "FileName"() -> (w1369:path)
                n813 = call <vilib>:"Check if File or Folder Exists.vi"("path"=w1369) -> ("file or folder exists?"=w1368:bool)  [unwired: 8 in, 2 out]
                n814 = case shown="True" w1368 {
                  tunnel: w1369 -> [_ w1374]
                  frame False {
                  }
                  frame True {
                    n815 = Strip Path(path=w1374) -> (name=w1373:string)  [unwired: 1 out]
                    n816 = Search and Replace String(input string=w1373, search string=".tmp", replace string=".csv" ("search string")) -> (result string=w1371:string, error out=w1377:errorcluster)  [unwired: 5 in, 2 out]
                    n817 = Build Path(base path="Save File Directory", name or relative path=w1371) -> (appended path=w1370:path)
                    n818 = local write "FileName"(w1370) -> ()
                    n819 = Move(source path=w1374, error in=w1377, 10:w1370) -> ()  [unwired: 2 in, 3 out]
                  }
                }
              }
              frame #5 {
                n820 = local read "Computer Name"() -> (w1378:string)
                n821 = local read "Ver."() -> (w1379:string)
                n822 = property class="App"() -> ("App.Name"=w1382:string)  [unwired: 2 in, 2 out]
                n823 = local read "LAN IP Address"() -> (w1383:string)
                n824 = call <vilib>:"Space Constant.vi"() -> ("String"=w1381:string)
                n825 = Concatenate Strings(w1383, w1381, w1378, w1381, w1382, w1381, w1379, w1381, "Completed." ("string")) -> (w1384:string)
                n826 = call "Save Time to File.vi"("String"=w1384) -> ()  [unwired: 13 in, 2 out]
              }
              frame #6 {
                n827 = global read "Global HEWH.vi" "Test Station:"() -> (w1386:string)
                n828 = Concatenate Strings("robocopy c:/Data //10.2.0.10/AP2Lab/" ("command line"), w1386) -> (w1385:string)
                n829 = call <vilib>:"System Exec.vi"("command line"=w1385) -> ()  [unwired: 7 in, 4 out]
              }
              frame #7 {
                n830 = event shown="[1] \"StopSerial\": Value Change" {
                  selector: _ -> [_ _]
                  dyn-events: _ -> [_ _]
                  timeout: _ -> [_ _]
                  event Timeout {
                    n831 = event-data() -> ()  [unwired: 1 in, 2 out]
                  }
                  event "StopSerial": Value Change {
                    w1388 = FALSE ("stop")
                    n832 = event-data() -> ()  [unwired: 1 in, 5 out]
                    n833 = local write "Stop Logging"(w1388) -> ()
                    n834 = property on="Stop Logging" class="Bool (strict)"("Val(Sgnl)"=w1388) -> ()  [unwired: 2 in, 2 out]
                    n835 = local write "STATUS"("Stopped OK" ("STATUS")) -> ()
                  }
                }
              }
            }
          }
        }
      }
      event "Help": Value Change {
        n836 = event-data() -> ()  [unwired: 1 in, 5 out]
        n837 = One Button Dialog(message="\n10 CFR part 430 5.1.4 First-Hour Rating Test\n5.1.4.3.P1.2\tWater heater not operating, initiate a draw\n5.1.4.3.P1.3\tTerminate draw after cut in of the upper most element\n5.1.4.3.P1.4\tAfter cut out, monitor 6 internal Tcs every minute\n5.1.4.3.P2.1\tInitiate draw After cut out and average tank temp is max\n5.1.4.3.P2.2\tRecord output water temp after 15 secs, and at 5 sec intervals thereafter\n5.1.4.3.P2.3\tMonitor inlet water temp, must be 58 +/- 2 F\n5.1.4.3.P2.4\tTerminate draw when ouytput temp = T*max -25F, record T*min\n5.1.4.3.P2.5\tRecord ave output water temp, Mass/volumt removed\n5.1.4.3.P3.1\tPerform second draw when eletricity to heating is reduced\n5.1.4.3.P4\tRepeat for 1 hour\n\tLast draw: there are special cases\n5.1.4.3.P5.1\tA  draw is going at t-1 hr, complete\n5.1.4.3.P5.1.5\tIf a draw is not going, immediately start and continue for at least 30 seconds\n5.1.4.3.P5.1.6\t If after 30 sec, T< last tmin, stop and discard measurements, else continue\n") -> (true=w1391:bool)  [unwired: 1 in]
        n838 = Not(x=w1391) -> (.not. x?=w1390:bool)
        n839 = local write "Help"(w1390) -> ()
      }
      event "Time Reset": Value Change {
        n840 = event-data() -> ()  [unwired: 1 in, 5 out]
        n841 = call "E-Time.vi"("Set Start Time (s)"="Time Update", "Reset"="Time Reset") -> ("error out"=w1393:errorcluster)  [unwired: 7 in, 2 out]
        n842 = flat-sequence {
          tunnel: w1393 -> [_]
          frame #0 {
            n843 = local write "Time Reset"(FALSE ("Time Reset")) -> ()
          }
        }
      }
      event Value Change {
        n844 = event-data() -> ()  [unwired: 1 in, 5 out]
        n845 = local read "Water Heater GEA2 Data"() -> (w1398:T1)
        n846 = local read "GEA2 HyperData"() -> (w1397:bool)
        n847 = local read "Use Agilent?"() -> (w1410:bool)
        n848 = local read "Label Array"() -> (w1409:string[])
        n849 = local read "Chanel List"() -> (w1414:string)
        n850 = local read "Equipment"() -> (w1412:T5)
        n851 = local read "Semiphore"() -> (w1413:T6)
        n852 = control-ref of="Tank Display"() -> (w1415:refnum<vi>)
        n853 = local read "FileName"() -> (w1402:path)
        n854 = local read "Calibration File Array"() -> (w1399:dbl[][])
        n855 = call "Gather Test Data - Heatup Test new.vi"("Power Analyzer"=w1414, "GEA2?"=w1413, "Equipment"=w1412, "WT210 Current"=w1397, "Tank Display Ref"=w1415, "MW100 TC Headers"=w1410, 9:"Calibration Coefficients"=w1399, 13:"Calibration Coefficients"=w1398, 14:w1409) -> ("Output Data"=w1408:string[][], "POWER"=→"POWER":T8, "Read Mass Flow Rate"=w1411:bool)  [unwired: 1 in, 3 out]
        n856 = local write "Voltage"(w1411) -> ()
        n857 = local write "Log Data"(w1408) -> ()
        n858 = Index Array(array=w1408, index (row)=1) -> (element=w1405:string[])  [unwired: 1 in]
        n859 = call-poly <vilib>:"Write To Spreadsheet File.vi"("delimiter (\\t)"="," ("delimiter (\\t)"), "append to file? (new file:F)"=TRUE, "1D data"=w1405, "file path (dialog if empty)"=w1402) -> ("new file path (Not A Path if cancelled)"=w1401:path)  [unwired: 4 in]
        n860 = call "Log String to Spreadsheet.vi"("String"="Power Change", "FileName"=w1401) -> ()  [unwired: 9 in, 1 out]
      }
    }
  }
  n861 = flat-sequence {
    tunnel: w12 -> [_]
    frame #0 {
      w1416 = TRUE ("stop")
      n862 = property on="stop" class="Bool (strict)"("Val(Sgnl)"=w1416) -> ()  [unwired: 2 in, 2 out]
      n863 = local write "stop"(w1416) -> ()
    }
  }
